vi "DB UI - Logon.vi"() -> ()   [LabVIEW 2013]
uses:
  Controls/Combo Box.ctl
  Controls/DB - Logon Extra Info.ctl
  Controls/DB - Logon Info.ctl
  <vilib>/Utility/miscctls.llb/LVComboBoxStrsAndValuesArrayTypeDef.ctl
  Controls/Logon - Enum.ctl
  Controls/DB - Logon Authentication Enum.ctl
  Controls/Global CMS.vi
  Controls/Global AMS.vi
  Controls/Global SRTRS.vi
  <vilib>/addons/database/Connection.llb/DB Tools Open Connec (String).vi
  <vilib>/addons/database/Connection.llb/Conn Execute.vi
  <vilib>/addons/database/Recordset.llb/Rec Fetch Recordset Data (R).vi
  <vilib>/addons/database/Recordset.llb/Rec Destroy - Connection.vi
  <vilib>/addons/database/Recordset.llb/Rec Fetch String Data (R).vi
  <vilib>/addons/database/NI_Database_API.lvlib
  <vilib>/Utility/miscctls.llb/LVPointTypeDef.ctl
panel:
  in  "Simulate DB Fail":bool
  out "DB available":bool
  in  "Main Application Directory (SRTRS/CMS/AMS)":path
  out "MHandler":errorcluster
  out "[IsUnicode]":bool[](array[boolean])
  out "User Has Access":bool
  out "[Stations]":string[](array[string])
  out "[AllStations]":bool
  in  "DB.Config.UserStationAccess":string="SRTRS.Config.UserStationAccess"
  out "2D data":string[][](array[string])
  in  "Overwrite HostName [ClientName] (Testing)":string
  out "Station Description":string
  out "[ClientName] Found":bool
  out "Logon":T1
  out "Logon Extra":T2
  out "Logon OK":bool
  out "[RawDataReport]":bool
  out "[TabUserAccess]":bool[](array[boolean])
  in  "Application":string
  out "DB Error":errorcluster
  out "[SpecialPrivilege] List":string[][](array[string])
  out "Logon Error":errorcluster
  in  "DB.Config.TabUserAccess":string="SRTRS.Config.TabUserAccess"
  out "[DefaultLanguage]":string
  in  "SRTRS.Config.System":string="SRTRS.Config.System"
  in  "Reinehold":bool
  out "[UserName]":string
  out "Logon PASS":bool
  in  "DB.Admin.Users":string="SRTRS.Admin.Users"
  in  "AD Simulate":T3(ring)=enum."Disable Simulation"
  out "Plant Description":string
  out "SQL":string[](array[string])
  out "[PlantId]":string
  out "[StationId]":string
  out "Initialize":bool
  out "Hostname [ClientName]":string
  in  "DB.Config.Parameter":string="SRTRS.Config.Parameter"
  in  "DB.Config.Plant":string="SRTRS.Config.Plant"
  out "Error Out":errorcluster
  in  "DB.Config.Language":string="SRTRS.Config.Language"
  in  "DB.Config.Domain":string="SRTRS.Config.Domain"
  in  "SRTRS.Config.StationSysRelation":string="SRTRS.Config.StationSysRelation"
  in  "DB.Config.Station":string="SRTRS.Config.Station"
  out "Connection Information":T4={"Connection "="SQL Server 32bit HPEnvy", "Username"="admin", "Password"="admin123"}
  out "AD available":bool
  out "Language (long form)":string
  in  "Logon Button":bool caption="Material New"
  in  "Station":T5
  in  "Plant":T5
  in  "Language":T5="English"
  in  "Domain":T5
  in  "Password":string
  in  "User":string
  # "Variables to be passed to calling VI (Must have same Label)"
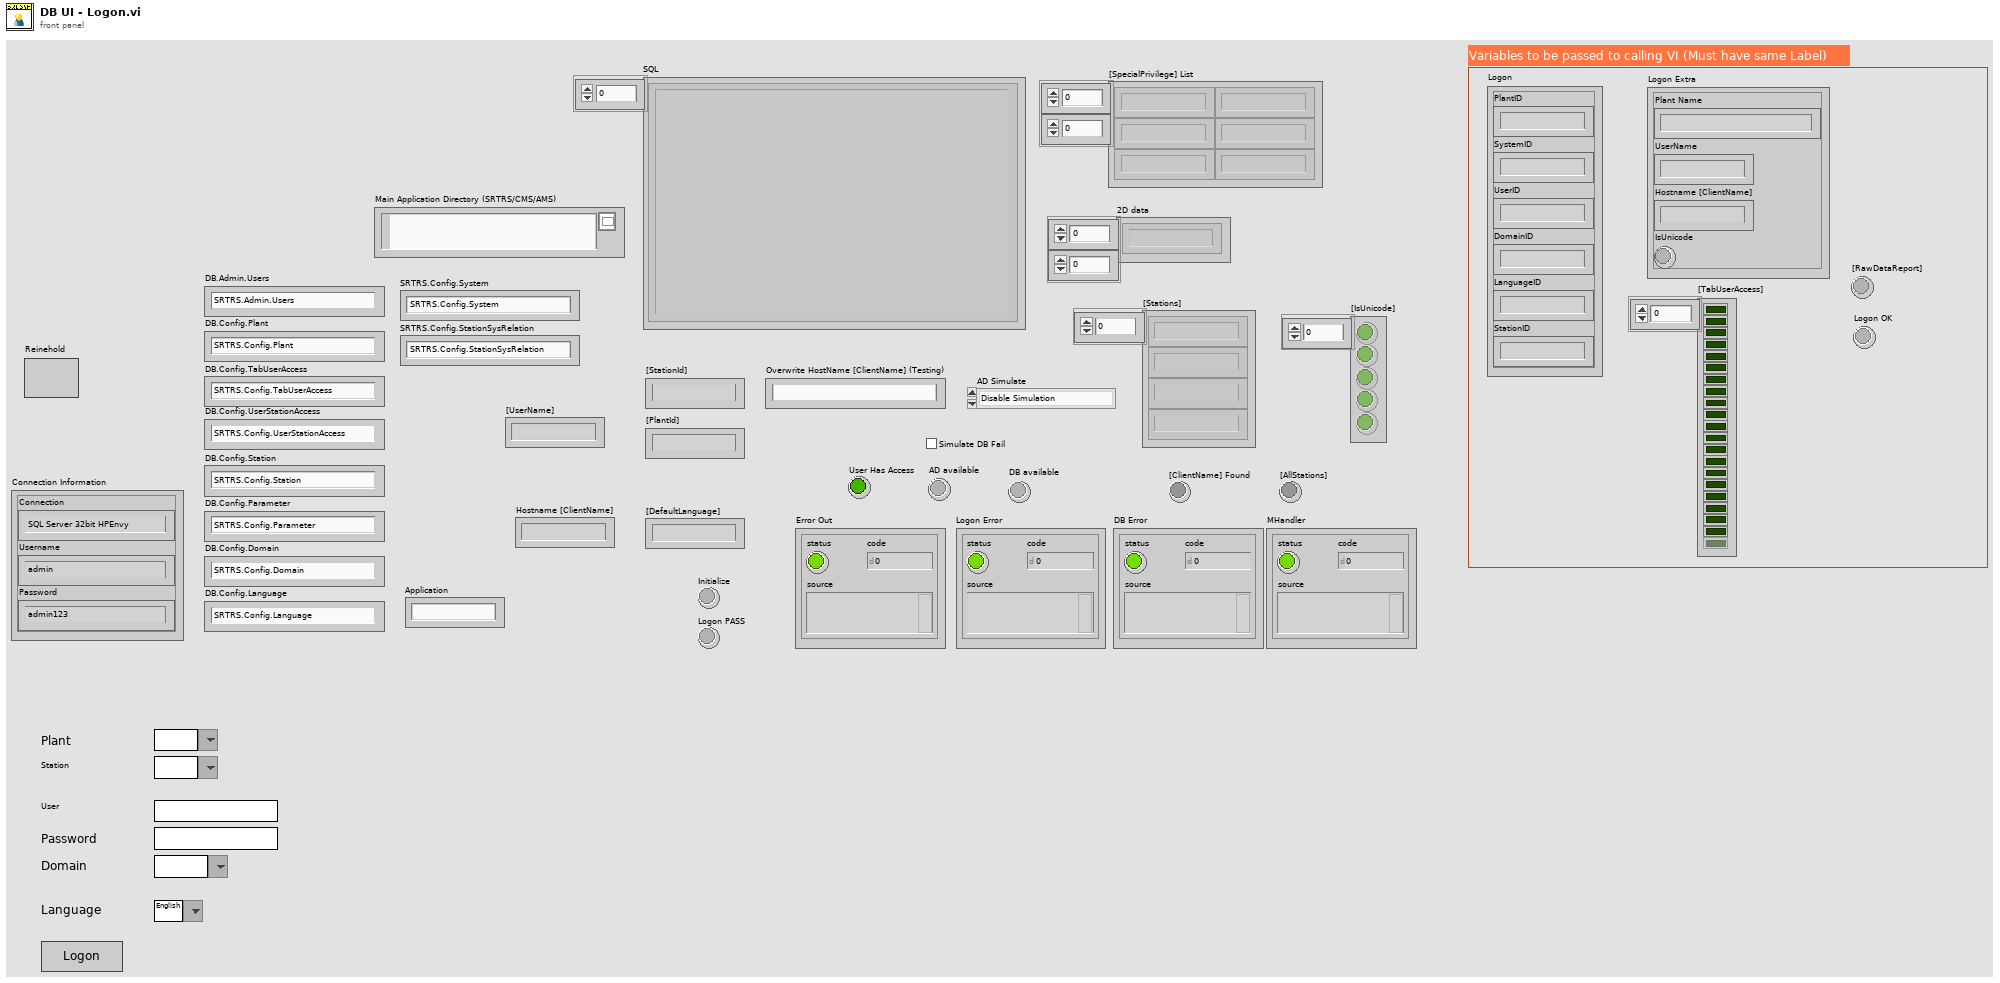
[diagram p1: front panel]
types:
  T1 = typedef "DB - Logon Info.ctl" = cluster{"PlantID":string, "SystemID":string, "UserID":string, "DomainID":string, "LanguageID":string, "StationID":string}
  T2 = typedef "DB - Logon Extra Info.ctl" = cluster{"Plant Name":string, "UserName":string, "Hostname [ClientName]":string, "IsUnicode":bool}
  T3 = enum16{"Simulate AD Available", "Simulate AD NOT Available", "Disable Simulation"}
  T4 = cluster{"Connection ":string, "Username":string, "Password":string}
  T5 = typedef "Combo Box.ctl" = string
  T6 = typedef "LVComboBoxStrsAndValuesArrayTypeDef.ctl" = cluster{"String":string, "Value":string}[]
  T7 = typedef "LVPointTypeDef.ctl" = cluster{"Horizontal":i16, "Vertical":i16}
  T8 = typedef "Connection Information Cluster.ctl" = cluster{"Connection ":string, "Username":string, "Password":string}
  T9 = typedef "NI_Database_API.lvlib/Conn ObjectReference.ctl" = refnum<k1>
  T10 = typedef "Logon - Enum.ctl" = enum16{"PC username", "PC username INFO", "Hostname", "Check AD", "Logon", "QUIT"}
  T11 = typedef "DB - Logon Authentication Enum.ctl" = enum16{"AD Authentication", "Local Authentication", "NO Authentication", "NODB Authentication"}
  T12 = typedef "DB - DB.Schema.Table.ctl" = cluster{"DB":string, "Schema":string, "Table":string}
  T13 = typedef "NI_Database_API.lvlib/Rec ObjectReference.ctl" = refnum<k1>
  T14 = cluster{"PC username":string, "Domain":string, "AD available":bool, "Username FOUND":bool, "Logon Full Name":string}
  T15 = typedef "eventvkey.ctl" = enum16{"ASCII", "Enter", "Return", "Shift", "Ctrl", "Alt", "Cmd", "Opt", "Caps", "NumLock", "Clear", "Break", "Up", "Down", "Left", "Right", "Insert", "Delete", "Home", "End", "PageUp", "PageDown", "Escape", "Help", "Pause", "ScrollLock", "F1", "F2", "F3", "F4", "F5", "F6", "F7", "F8", "F9", "F10", "F11", "F12", "F13", "F14", "F15", "F16", "F17", "F18", "F19", "F20", "F21", "F22", "F23", "F24", "Play", "VolumeUp", "VolumeDown", "Mute", "Two Byte Char"}
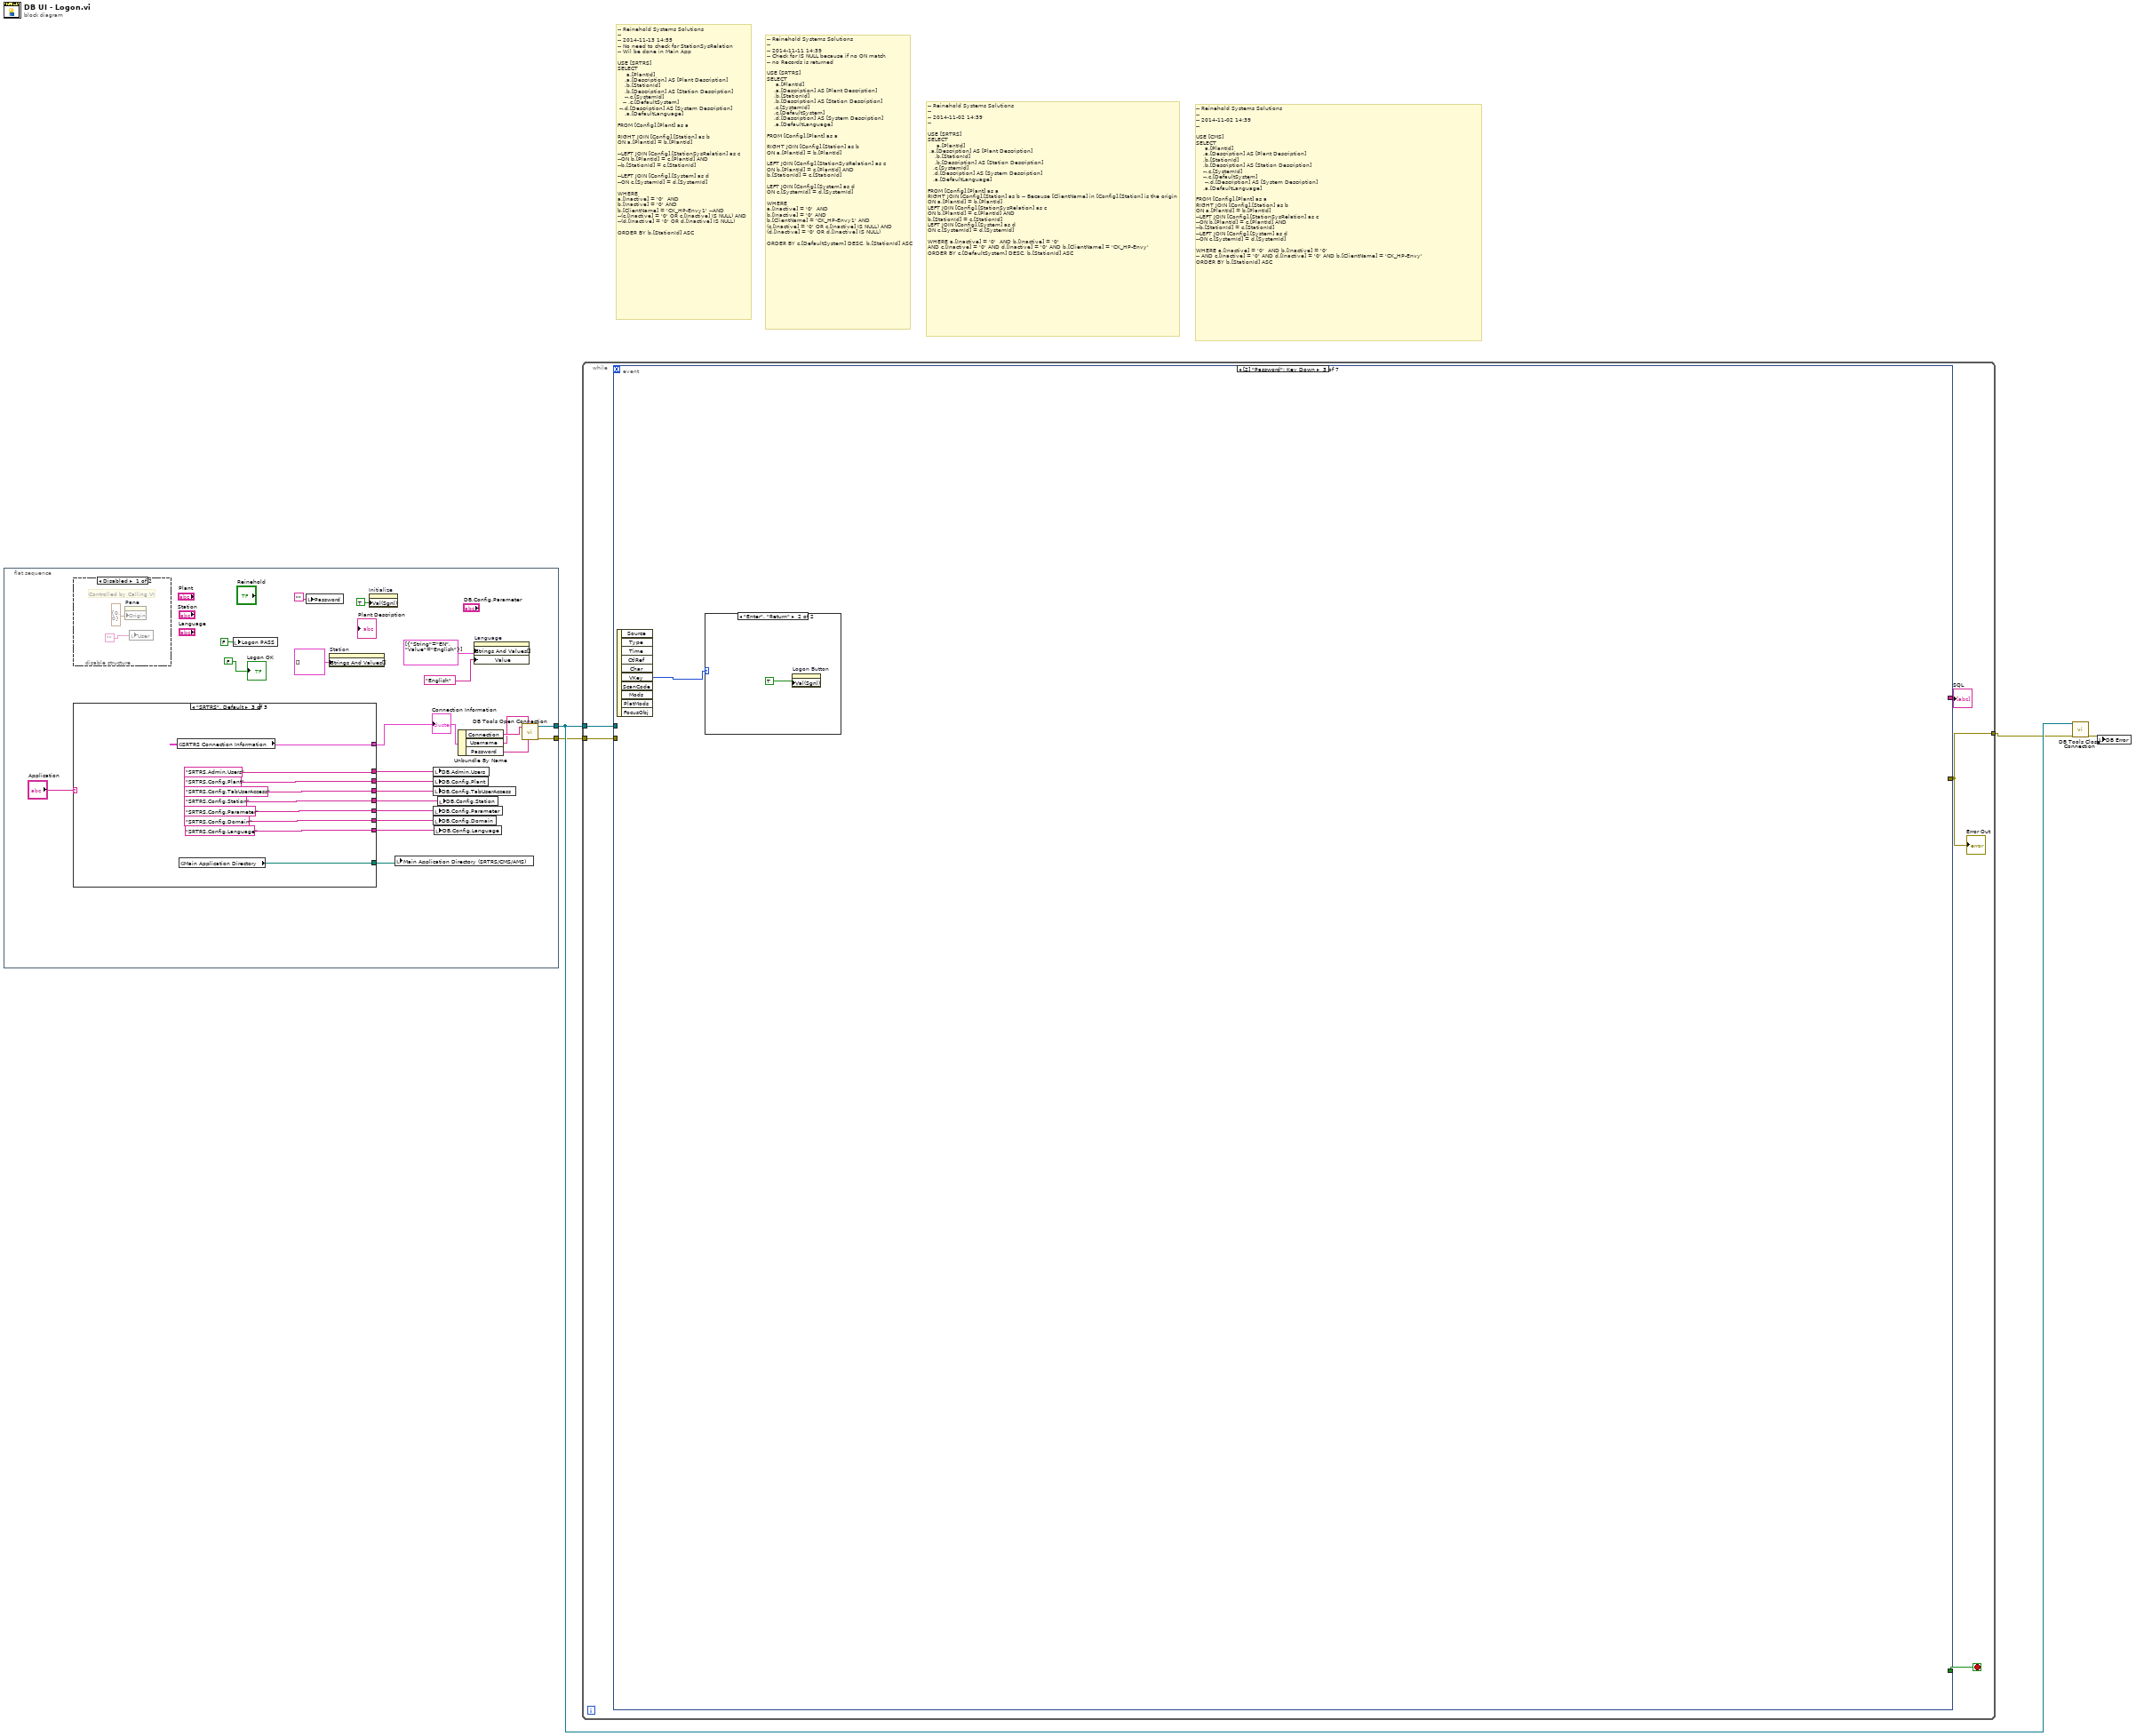
[diagram p0: block diagram]
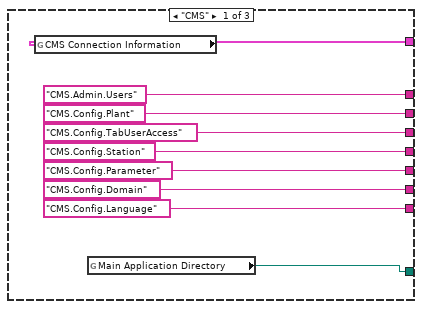
[diagram p3: hidden frame]
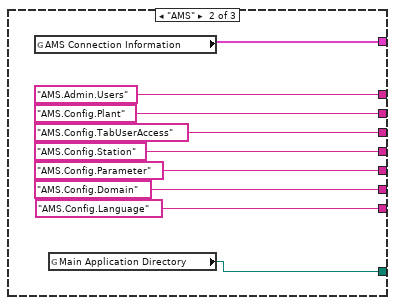
[diagram p4: hidden frame]
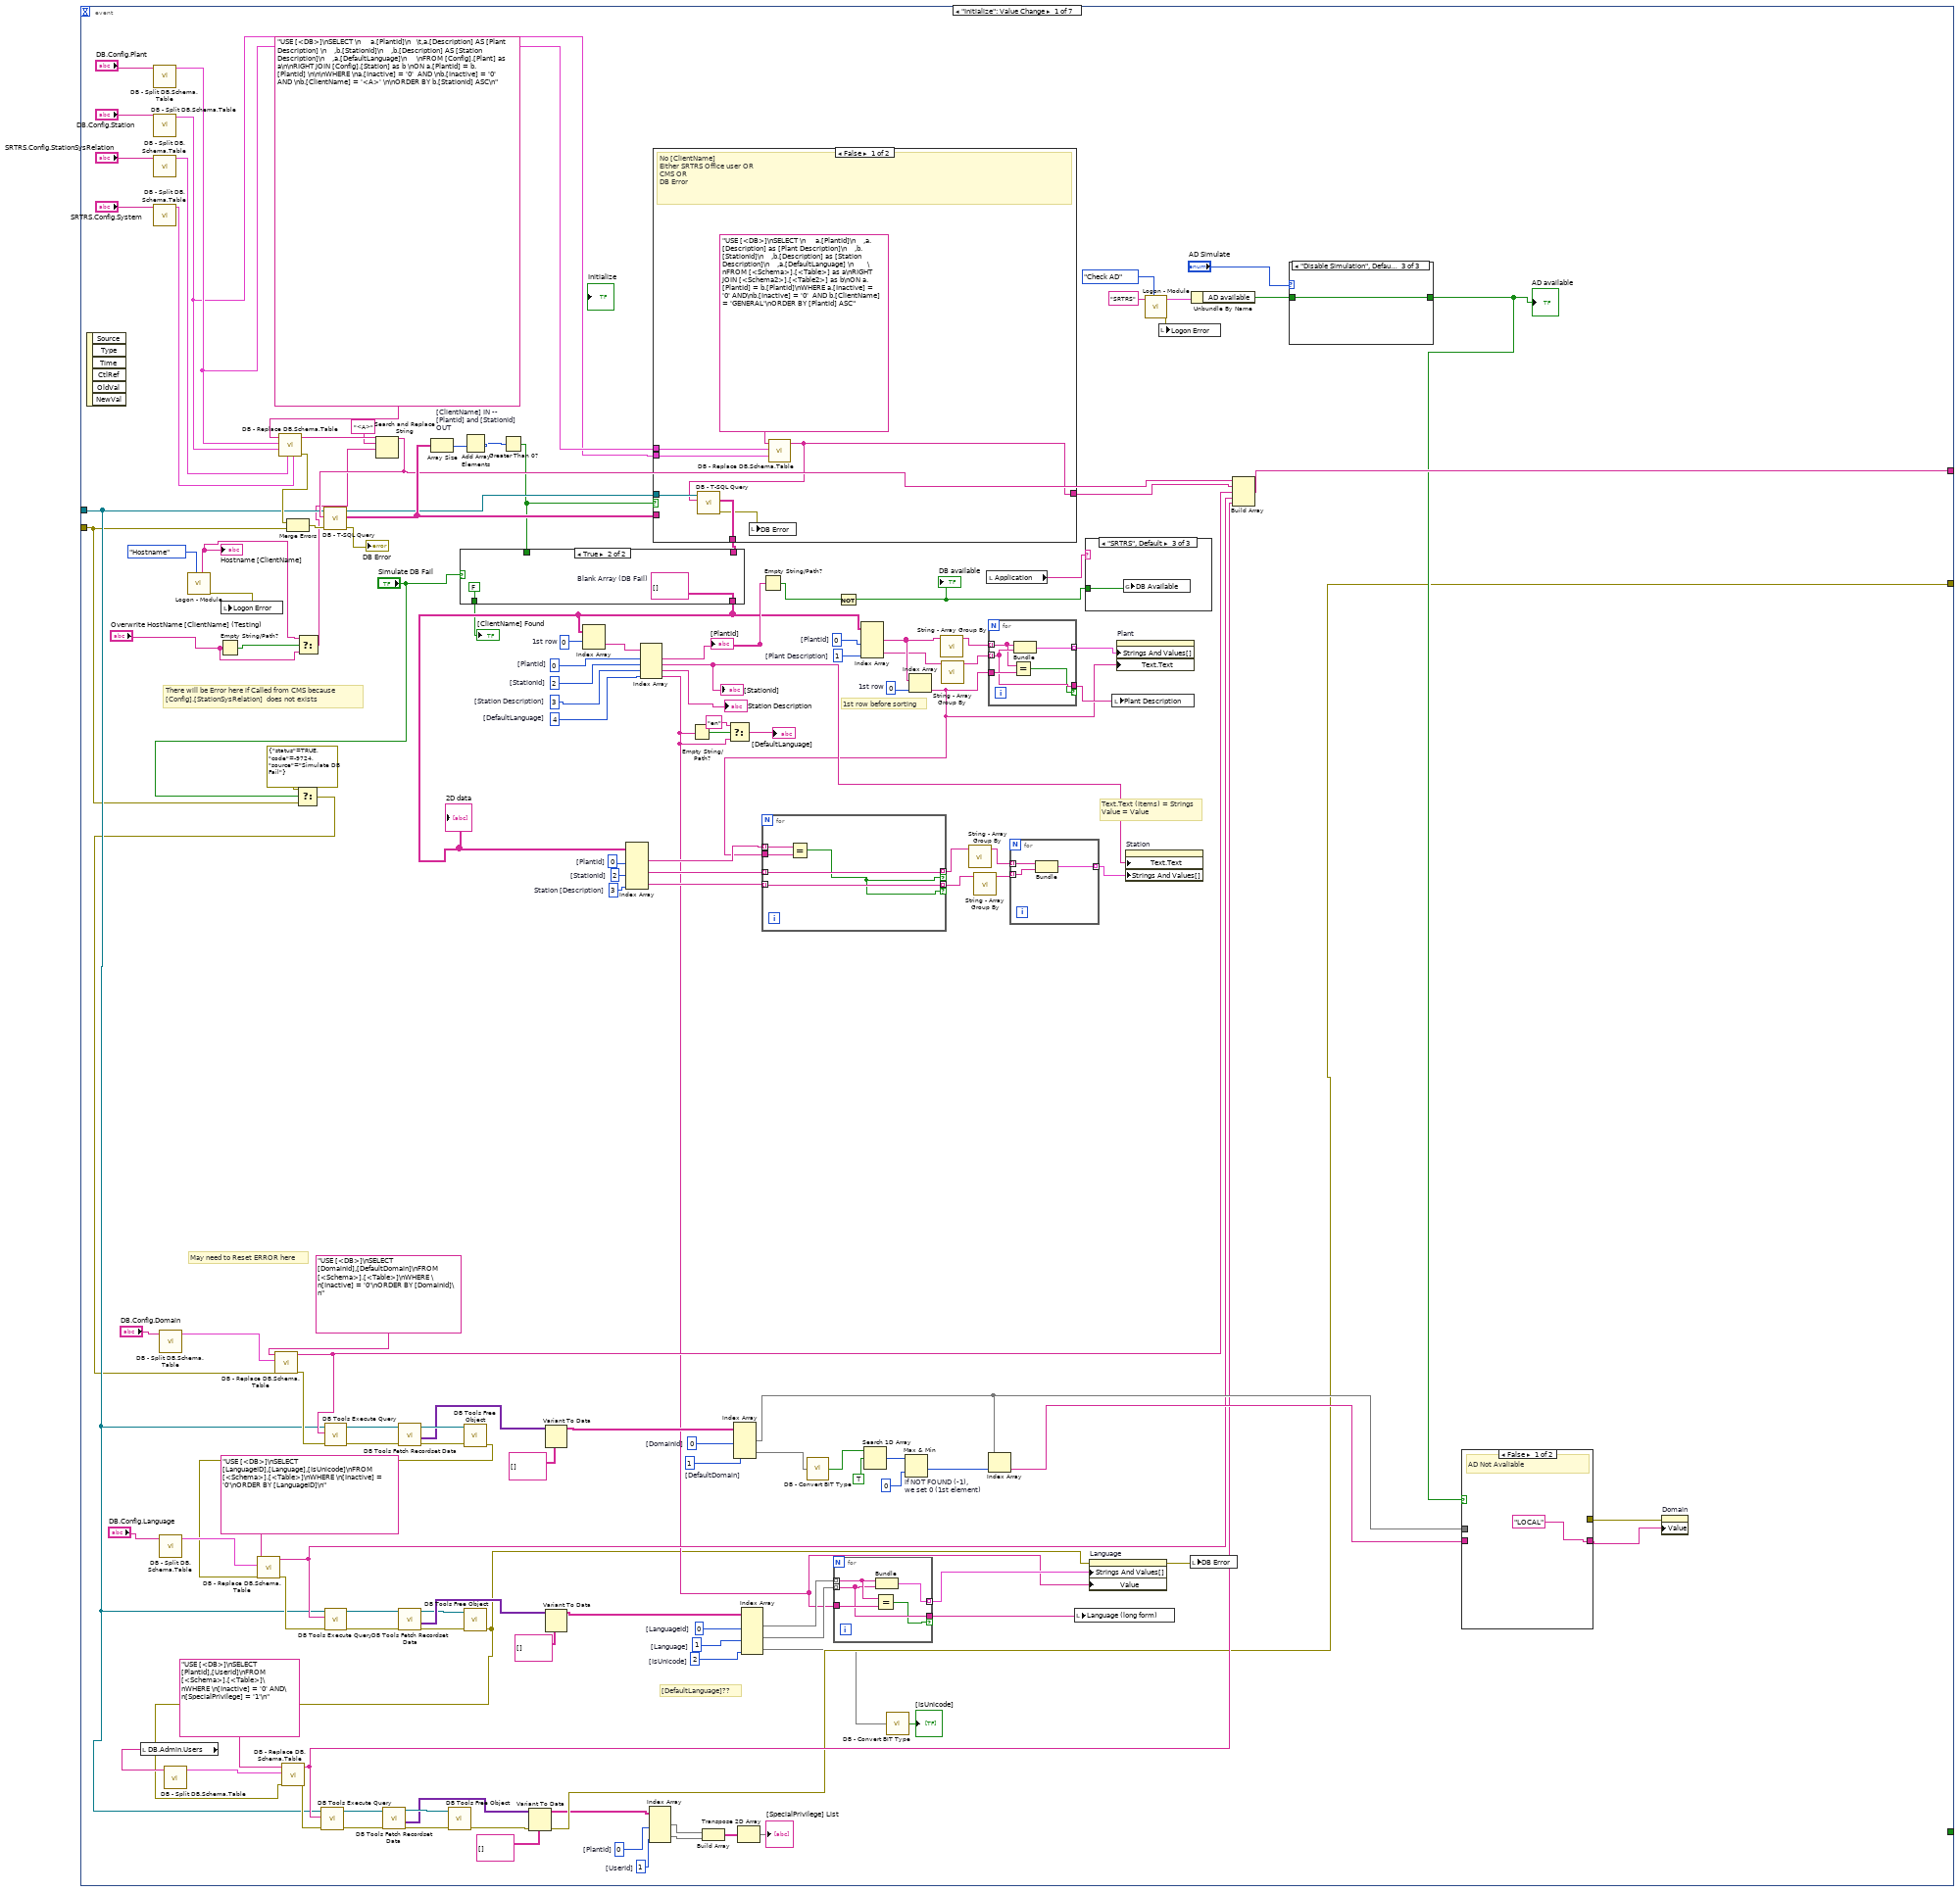
[diagram p5: hidden frame]
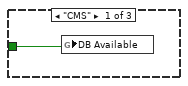
[diagram p7: hidden frame]
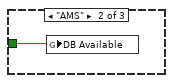
[diagram p8: hidden frame]
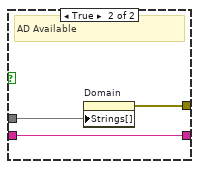
[diagram p10: hidden frame]
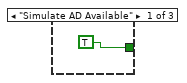
[diagram p11: hidden frame]
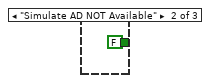
[diagram p12: hidden frame]
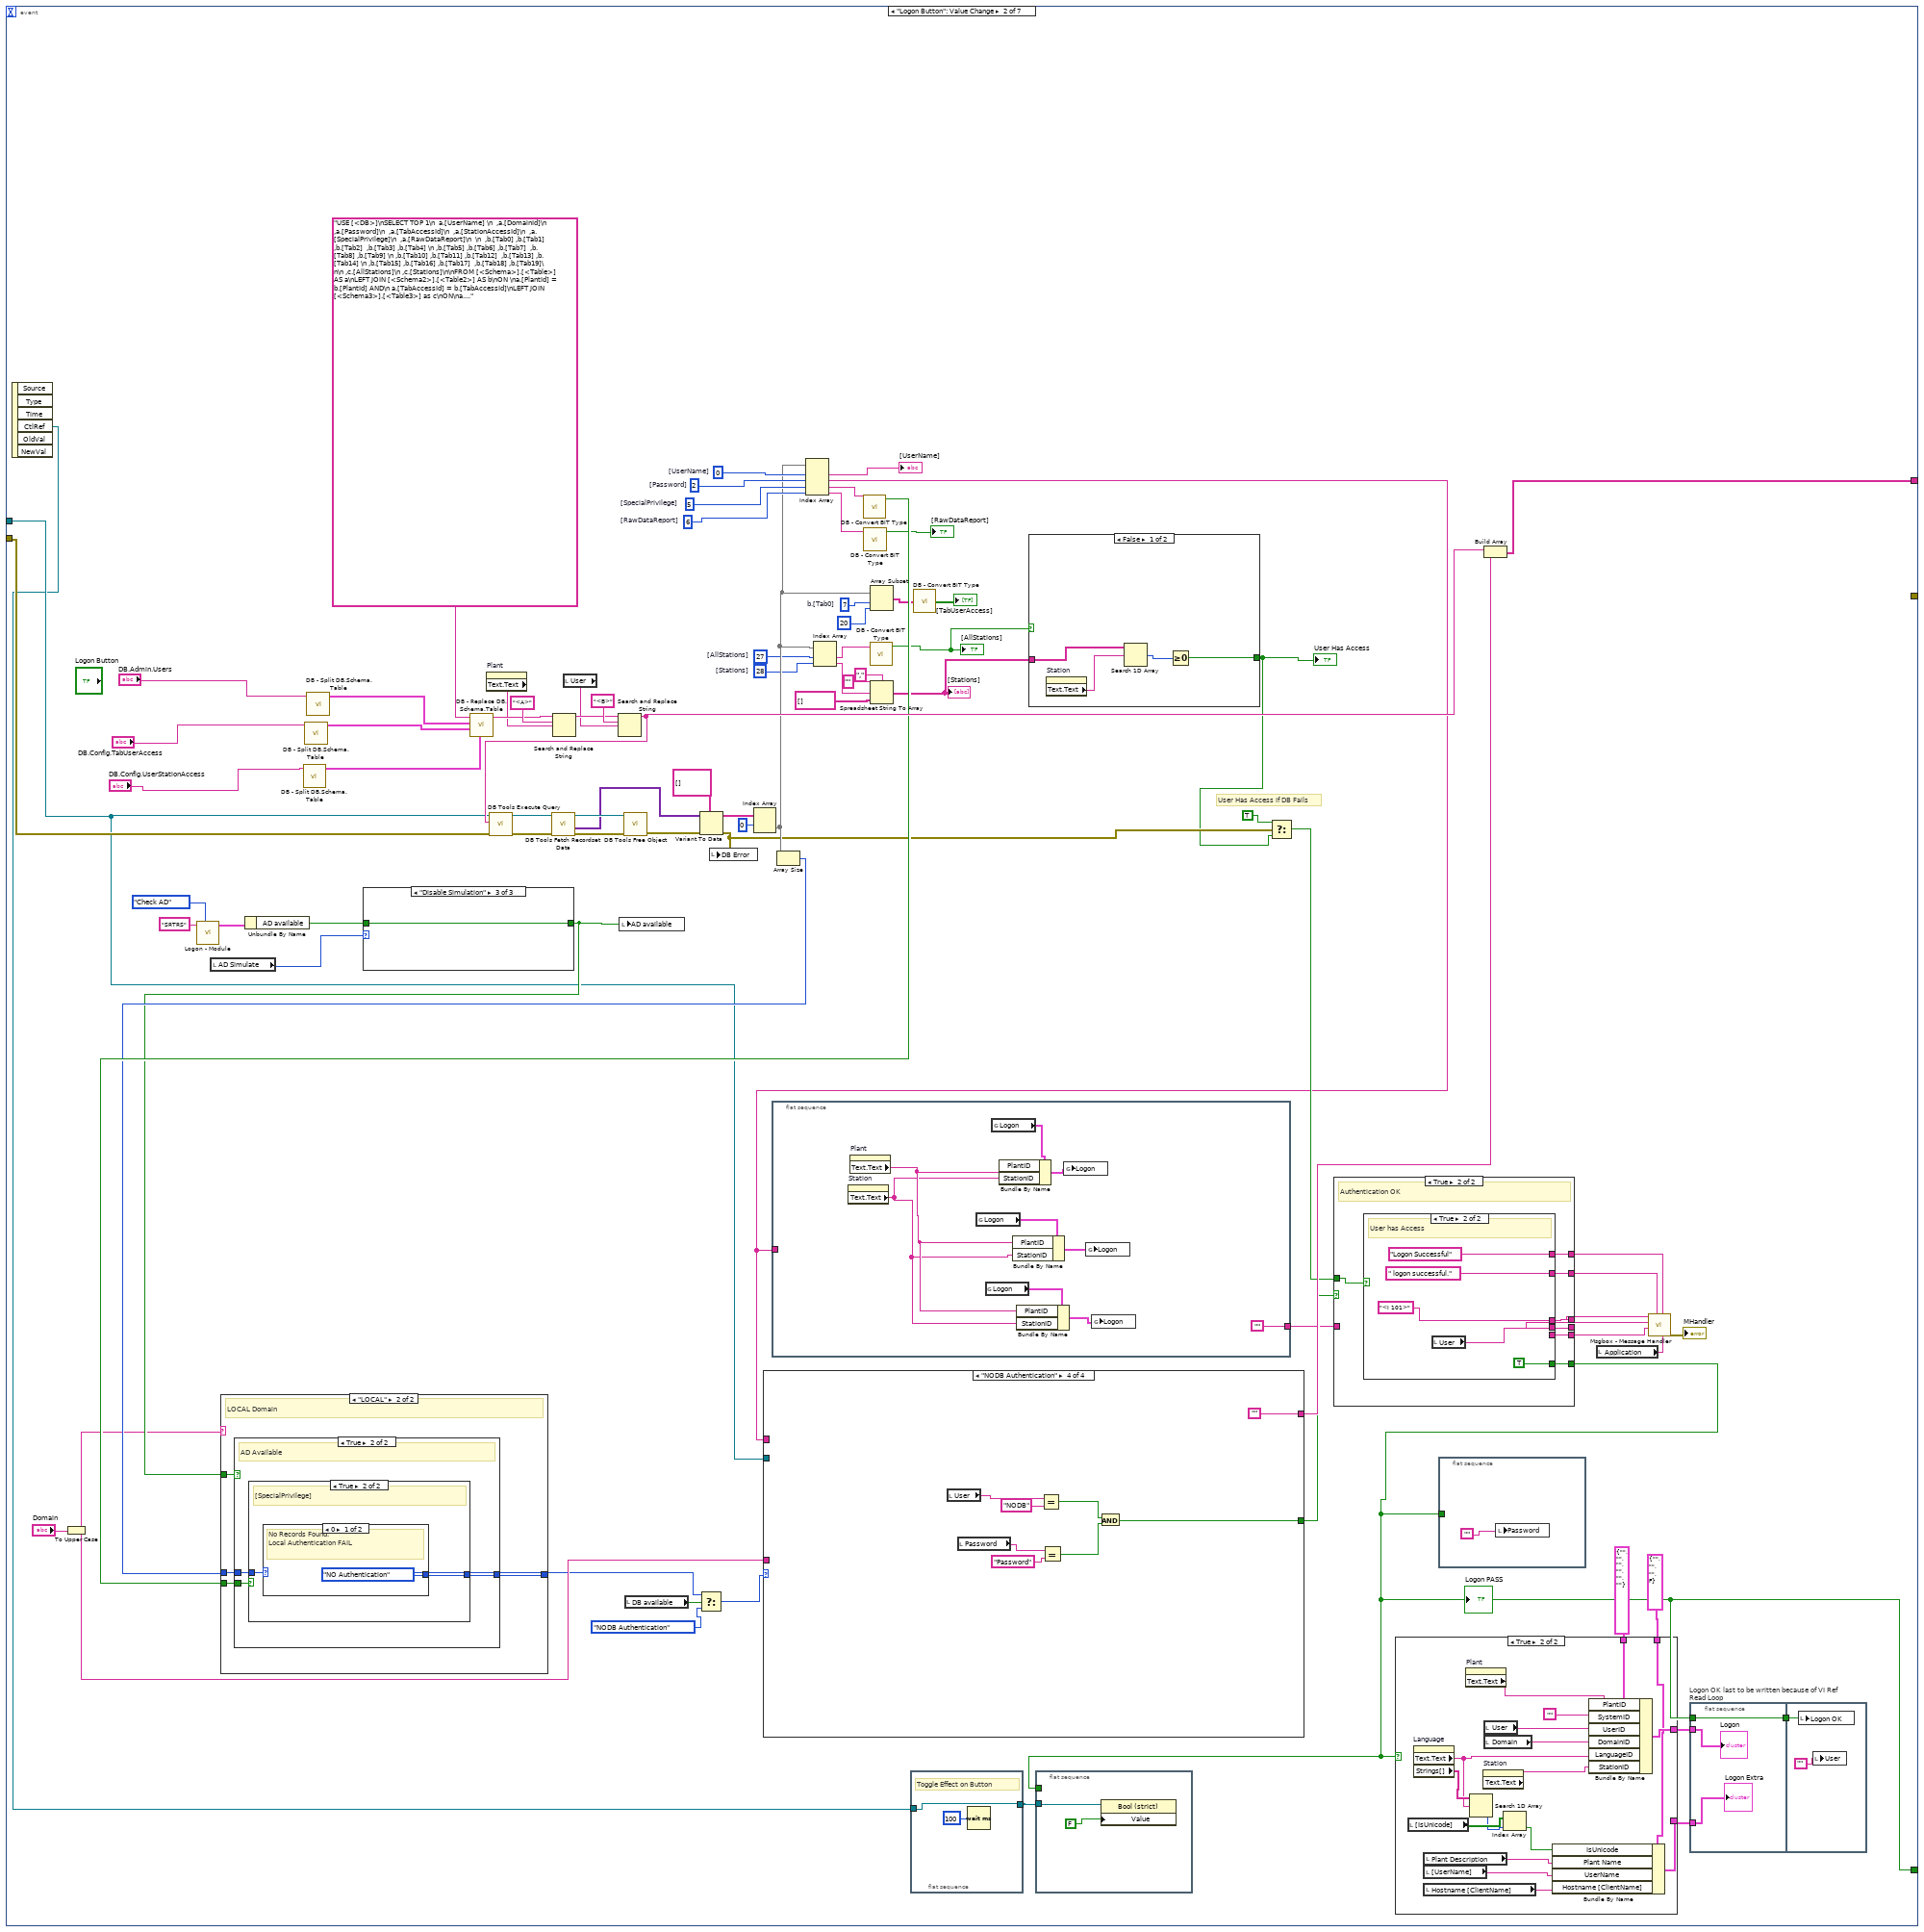
[diagram p13: hidden frame]
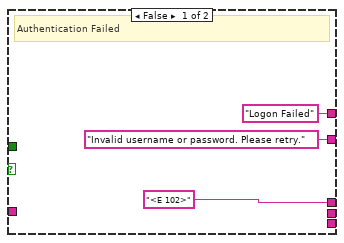
[diagram p14: hidden frame]
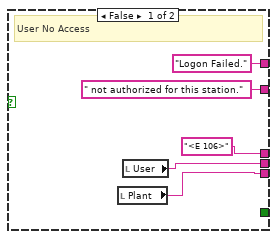
[diagram p15: hidden frame]
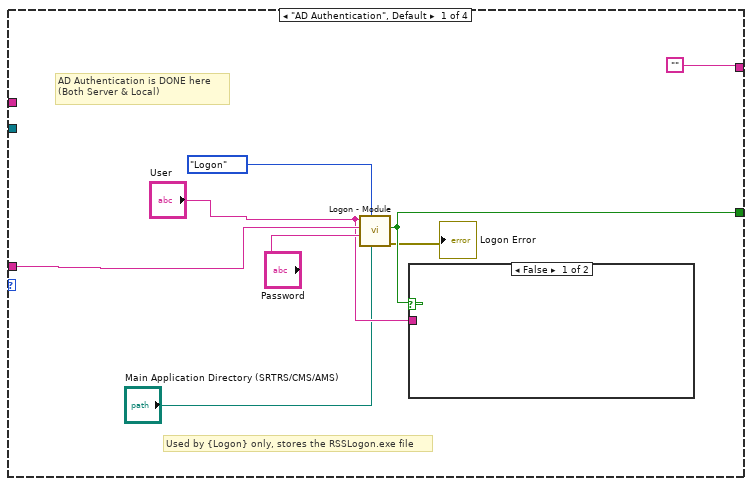
[diagram p18: hidden frame]
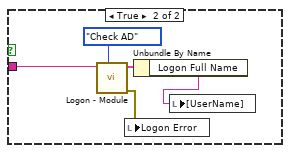
[diagram p19: hidden frame]
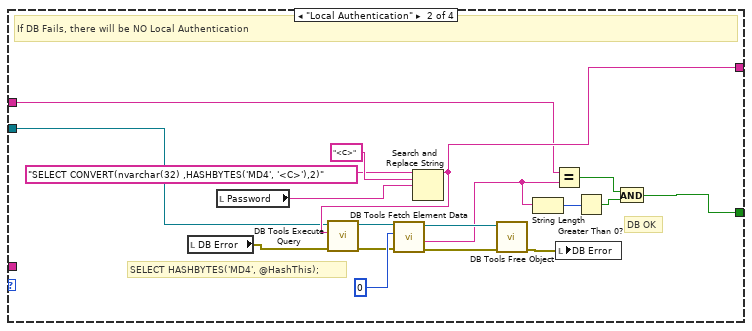
[diagram p20: hidden frame]
diagram:
  # "-- Reinehold Systems Solutions\n--\n-- 2014-11-13 14:55\n-- No need to check for StationSysRelation\n-- Wil be done in Main App\n\nUSE [SRTRS]\nSELECT \n     a.[PlantId]\n   \t,a.[Description] AS [Plant Description] \n    ,b.[StationId]\n    ,b.[Description] AS [Station Description]\n   \t--,c.[SystemId]\n   -- ,c.[DefaultSystem]\n\t--,d.[Description] AS [System Description]\n    ,a.[DefaultLanguage]\n     \nFROM [Config].[Plant] as a\n\nRIGHT JOIN [Config].[Station] as b \nON a.[PlantId] = b.[PlantId] \n\n--LEFT JOIN [Config].[StationSysRelation] as c\n--ON b.[PlantId] = c.[PlantId] AND\n--b.[StationId] = c.[StationId] \n\n--LEFT JOIN [Config].[System] as d\n--ON c.[SystemId] = d.[SystemId] \n \nWHERE \na.[Inactive] = '0'  AND \nb.[Inactive] = '0' AND \nb.[ClientName] = 'CK_HP-Envy1' --AND\n--(c.[Inactive] = '0' OR c.[Inactive] IS NULL) AND \n--(d.[Inactive] = '0' OR d.[Inactive] IS NULL)  \n\nORDER BY b.[StationId] ASC"
  # "-- Reinehold Systems Solutions\n--\n-- 2014-11-11 14:39\n-- Check for IS NULL because if no ON match\n-- no Records is returned\n\nUSE [SRTRS]\nSELECT \n     a.[PlantId]\n   \t,a.[Description] AS [Plant Description] \n    ,b.[StationId]\n    ,b.[Description] AS [Station Description]\n   \t,c.[SystemId]\n    ,c.[DefaultSystem]\n\t   ,d.[Description] AS [System Description]\n    ,a.[DefaultLanguage]\n     \nFROM [Config].[Plant] as a\n\nRIGHT JOIN [Config].[Station] as b \nON a.[PlantId] = b.[PlantId] \n\nLEFT JOIN [Config].[StationSysRelation] as c\nON b.[PlantId] = c.[PlantId] AND\nb.[StationId] = c.[StationId] \n\nLEFT JOIN [Config].[System] as d\nON c.[SystemId] = d.[SystemId] \n \nWHERE \na.[Inactive] = '0'  AND \nb.[Inactive] = '0' AND \nb.[ClientName] = 'CK_HP-Envy1' AND\n(c.[Inactive] = '0' OR c.[Inactive] IS NULL) AND \n(d.[Inactive] = '0' OR d.[Inactive] IS NULL)  \n\nORDER BY c.[DefaultSystem] DESC, b.[StationId] ASC"
  # "-- Reinehold Systems Solutions\n--\n-- 2014-11-02 14:39\n--\n\nUSE [CMS]\nSELECT \n     a.[PlantId]\n   \t,a.[Description] AS [Plant Description] \n    ,b.[StationId]\n    ,b.[Description] AS [Station Description]\n   \t--,c.[SystemId]\n    --,c.[DefaultSystem]\n\t    --,d.[Description] AS [System Description]\n    ,a.[DefaultLanguage]\n\nFROM [Config].[Plant] as a\nRIGHT JOIN [Config].[Station] as b \nON a.[PlantId] = b.[PlantId]\n--LEFT JOIN [Config].[StationSysRelation] as c\n--ON b.[PlantId] = c.[PlantId] AND\n--b.[StationId] = c.[StationId]\n--LEFT JOIN [Config].[System] as d\n--ON c.[SystemId] = d.[SystemId]\n\nWHERE a.[Inactive] = '0'  AND b.[Inactive] = '0' \n-- AND c.[Inactive] = '0' AND d.[Inactive] = '0' AND b.[ClientName] = 'CK_HP-Envy'\nORDER BY b.[StationId] ASC"
  # "-- Reinehold Systems Solutions\n--\n-- 2014-11-02 14:39\n--\n\nUSE [SRTRS]\nSELECT \n     a.[PlantId]\n\t,a.[Description] AS [Plant Description] \n    ,b.[StationId]\n    ,b.[Description] AS [Station Description]\n  \t,c.[SystemId]\n  \t,d.[Description] AS [System Description]\n   ,a.[DefaultLanguage]\n     \nFROM [Config].[Plant] as a\nRIGHT JOIN [Config].[Station] as b -- Because [ClientName] in [Config].[Station] is the origin\nON a.[PlantId] = b.[PlantId]\nLEFT JOIN [Config].[StationSysRelation] as c\nON b.[PlantId] = c.[PlantId] AND\nb.[StationId] = c.[StationId]\nLEFT JOIN [Config].[System] as d\nON c.[SystemId] = d.[SystemId]\n \nWHERE a.[Inactive] = '0'  AND b.[Inactive] = '0' \nAND c.[Inactive] = '0' AND d.[Inactive] = '0' AND b.[ClientName] = 'CK_HP-Envy'\nORDER BY c.[DefaultSystem] DESC, b.[StationId] ASC"
  n1 = flat-sequence {
    tunnel: [w23] -> w4
    tunnel: [w7] -> w3
    frame #0 {
      n2 = case shown="\"SRTRS\", Default" "Application" {
        tunnel: [w37 w39 w55] -> w19
        tunnel: ["CMS.Admin.Users" ("DB.Schema.Table\n(SRTRS.Admin.Users)") "AMS.Admin.Users" ("DB.Schema.Table\n(SRTRS.Admin.Users)") "SRTRS.Admin.Users" ("DB.Schema.Table\n(SRTRS.Admin.Users)")] -> w18
        tunnel: ["CMS.Config.Plant" ("DB.Schema.Table\nDB.Config.Plant") "AMS.Config.Plant" ("DB.Schema.Table\nDB.Config.Plant") "SRTRS.Config.Plant" ("DB.Schema.Table\nDB.Config.Plant")] -> w17
        tunnel: ["CMS.Config.TabUserAccess" ("DB.Config.TabUserAccess") "AMS.Config.TabUserAccess" ("DB.Config.TabUserAccess") "SRTRS.Config.TabUserAccess" ("DB.Config.TabUserAccess")] -> w16
        tunnel: ["CMS.Config.Station" ("SRTRS.Config.Station") "AMS.Config.Station" ("SRTRS.Config.Station") "SRTRS.Config.Station" ("SRTRS.Config.Station")] -> w15
        tunnel: ["CMS.Config.Parameter" ("DB.Config.Parameter") "AMS.Config.Parameter" ("DB.Config.Parameter") "SRTRS.Config.Parameter" ("DB.Config.Parameter")] -> w14
        tunnel: ["CMS.Config.Domain" ("DB.Config.Domain") "AMS.Config.Domain" ("DB.Config.Domain") "SRTRS.Config.Domain" ("DB.Config.Domain")] -> w13
        tunnel: ["CMS.Config.Language" ("DB.Config.TabUserAccess") "AMS.Config.Language" ("DB.Config.TabUserAccess") "SRTRS.Config.Language" ("DB.Config.TabUserAccess")] -> w12
        tunnel: [w29 w38 w47] -> w8
        frame "CMS" {
          n3 = global read "Global CMS.vi" "CMS Connection Information"() -> (w37:T8)
          n4 = global read "Global CMS.vi" "Main Application Directory"() -> (w29:path)
        }
        frame "AMS" {
          n5 = global read "Global AMS.vi" "AMS Connection Information"() -> (w39:T8)
          n6 = global read "Global AMS.vi" "Main Application Directory"() -> (w38:path)
        }
        frame "SRTRS", Default {
          n7 = global read "Global SRTRS.vi" "SRTRS Connection Information"() -> (w55:T8)
          n8 = global read "Global SRTRS.vi" "Main Application Directory"() -> (w47:path)
        }
      }
      "Connection Information" <- w19
      n9 = disable-structure shown="Disabled" {
        frame Disabled {
          # "Controlled by Calling VI"
          n10 = property on="Pane" class="Pane"("Origin"=T7 {"Horizontal"=0, "Vertical"=0}) -> ()  [unwired: 2 in, 2 out]
          n11 = local write "User"("") -> ()
        }
        frame Enabled {
        }
      }
      n12 = local write "Logon PASS"(FALSE ("Logon PASS")) -> ()
      n13 = local write "Password"("") -> ()
      n14 = property on="Station" class="CmbBox (strict)"("Strings And Values[]"=T6 [] ("Strings And Values []")) -> ()  [unwired: 2 in, 2 out]
      n15 = property on="Initialize" class="Bool (strict)"("Val(Sgnl)"=TRUE ("Value (Signaling)")) -> ()  [unwired: 2 in, 2 out]
      n16 = local write "Main Application Directory (SRTRS/CMS/AMS)"(w8) -> ()
      n17 = local write "DB.Admin.Users"(w18) -> ()
      n18 = local write "DB.Config.Plant"(w17) -> ()
      n19 = local write "DB.Config.TabUserAccess"(w16) -> ()
      n20 = local write "DB.Config.Parameter"(w14) -> ()
      n21 = local write "DB.Config.Domain"(w13) -> ()
      n22 = local write "DB.Config.Language"(w12) -> ()
      n23 = local write "DB.Config.Station"(w15) -> ()
      n24 = Unbundle By Name(w19) -> ("Connection"=w26:string, "Username"=w25:string, "Password"=w24:string)
      n25 = property on="Language" class="CmbBox (strict)"("Strings And Values[]"=T6 [{"String"="EN", "Value"="English"}] ("Strings And Values []"), "Value"=T5 "English" ("Language")) -> ()  [unwired: 2 in, 2 out]
      n26 = call-poly <vilib>:"DB Tools Open Connection.vi"("password"=w24, "userID"=w25, "connection information"=w26) -> ("error out"=w7:errorcluster, "connection reference"=w23:T9)  [unwired: 5 in]
      "Logon OK" <- FALSE ("Logon OK")
    }
  }
  n27 = while {
    tunnel: w4 -> [w59]
    tunnel: w3 -> [w58]
    tunnel: [w57] -> w2
    stop <- w60 stop-if-true
    n28 = event shown="[2] \"Password\": Key Down" {
      selector: _ -> [_ _ _ _ _ _ _]
      dyn-events: _ -> [_ _ _ _ _ _ _]
      timeout: _ -> [_ _ _ _ _ _ _]
      tunnel: [_ w259 _ _ _ _ _] -> w60
      tunnel: w59 -> [w101 w300 _ _ _ _ _]
      tunnel: w58 -> [w64 w320 _ _ _ _ _]
      tunnel: [w139 _ _ _ _ _ _] -> w57
      tunnel: [w202 w311 _ _ _ _ _] -> w56
      event "Initialize": Value Change {
        w81 = 2  # [IsUnicode]
        w84 = 0  # [PlantId]
        w93 = 3  # Station [Description]
        w99 = 2  # [StationId]
        w115 = 0  # 1st row
        w110 = 1  # [Plant Description]
        w109 = 0  # [PlantId]
        w135 = 1  # [UserId]
        w136 = 0  # [PlantId]
        w149 = 4  # [DefaultLanguage]
        w153 = 0  # 1st row
        w150 = 3  # [Station Description]
        w169 = 1  # [Language]
        w172 = 0  # [LanguageId]
        w192 = 1  # [DefaultDomain]
        w191 = 0  # [DomainId]
        w151 = 2  # [StationId]
        w152 = 0  # [PlantId]
        w208 = "USE [<DB>]\nSELECT \n     a.[PlantId]\n   \t,a.[Description] AS [Plant Description] \n    ,b.[StationId]\n    ,b.[Description] AS [Station Description]\n    ,a.[DefaultLanguage]\n     \nFROM [Config].[Plant] as a\n\nRIGHT JOIN [Config].[Station] as b \nON a.[PlantId] = b.[PlantId] \n\n\nWHERE \na.[Inactive] = '0'  AND \nb.[Inactive] = '0' AND \nb.[ClientName] = '<A>' \n\nORDER BY b.[StationId] ASC\n"  # [ClientName] IN --  [PlantId] and [StationId] OUT
        # "There will be Error here if Called from CMS because \n[Config].[StationSysRelation]  does not exists"
        # "1st row before sorting"
        # "May need to Reset ERROR here"
        # "Text.Text (Items) = Strings\nValue = Value"
        # "[DefaultLanguage]??"
        n29 = event-data() -> ()  [unwired: 1 in, 6 out]
        n30 = local read "DB.Admin.Users"() -> (w148:string)
        n31 = call "DB - Split DB.Schema.Table.vi"("DB.Schema.Table"="DB.Config.Plant") -> ("DB.Schema.Table"=w105:T12)  [unwired: 10 in]
        n32 = call "DB - Split DB.Schema.Table.vi"("DB.Schema.Table"="DB.Config.Station") -> ("DB.Schema.Table"=w104:T12)  [unwired: 10 in]
        n33 = call "DB - Split DB.Schema.Table.vi"("DB.Schema.Table"="SRTRS.Config.StationSysRelation") -> ("DB.Schema.Table"=w103:T12)  [unwired: 10 in]
        n34 = call "DB - Split DB.Schema.Table.vi"("DB.Schema.Table"="SRTRS.Config.System") -> ("DB.Schema.Table"=w102:T12)  [unwired: 10 in]
        n35 = call "DB - Split DB.Schema.Table.vi"("DB.Schema.Table"="DB.Config.Domain") -> ("DB.Schema.Table"=w198:T12)  [unwired: 10 in]
        n36 = call "DB - Split DB.Schema.Table.vi"("DB.Schema.Table"="DB.Config.Language") -> ("DB.Schema.Table"=w173:T12)  [unwired: 10 in]
        n37 = call "DB - Split DB.Schema.Table.vi"("DB.Schema.Table"=w148) -> ("DB.Schema.Table"=w146:T12)  [unwired: 10 in]
        n38 = call "Logon - Module.vi"("Logon - Enum"=Logon_-_Enum."Hostname") -> ("Error Out"=w129:errorcluster, "Hostname"=w96:string)  [unwired: 5 in, 4 out]
        "Hostname [ClientName]" <- w96
        n39 = Empty String/Path?(string/path="Overwrite HostName [ClientName] (Testing)") -> (empty?=w97:bool)
        n40 = local write "Logon Error"(w129) -> ()
        n41 = call "DB - Replace DB.Schema.Table.vi"("DB.Schema.Table 4"=w102, "DB.Schema.Table 3"=w103, "DB.Schema.Table 2"=w104, "DB.Schema.Table"=w105, "string in"=w208) -> ("error out"=w117:errorcluster, "string out"=w207:string)  [unwired: 5 in]
        n42 = Merge Errors(w117, w64) -> (w116:errorcluster)
        n43 = Select(t=errorcluster {"status"=TRUE, "code"=-9724, "source"="Simulate DB Fail"} ("error constant"), s="Simulate DB Fail", f=w64) -> (s? t:f=w65:errorcluster)
        n44 = call "DB - Replace DB.Schema.Table.vi"("error in (no error)"=w65, "DB.Schema.Table"=w198, "string in"="USE [<DB>]\nSELECT [DomainId],[DefaultDomain]\nFROM [<Schema>].[<Table>]\nWHERE \n[Inactive] = '0'\nORDER BY [DomainId]\n") -> ("error out"=w122:errorcluster, "string out"=w154:string)  [unwired: 7 in]
        n45 = Select(t=w96, s=w97, f="Overwrite HostName [ClientName] (Testing)") -> (s? t:f=w94:string)
        n46 = call-poly <vilib>:"DB Tools Execute Query.vi"("error in (no error)"=w122, "SQL query"=w154, "connection reference"=w101) -> ("error out"=w196:errorcluster, "recordset reference"=w201:T13)  [unwired: 5 in]
        n47 = Search and Replace String(input string=w207, search string="<A>" ("input string"), replace string=w94) -> (result string=w123:string)  [unwired: 5 in, 3 out]
        n48 = call "DB - T-SQL Query.vi"("error in (no error)"=w116, "T-SQL"=w123, "connection reference"=w101) -> ("error out"=→"DB Error":errorcluster, "2D data"=w126:string[][], "connection reference"=w125:T9)  [unwired: 6 in]
        n49 = call-poly <vilib>:"DB Tools Fetch Recordset Data.vi"("error in (no error)"=w196, "recordset reference"=w201) -> ("error out"=w195:errorcluster, "recordset data"=w193:variant[][], "recordset reference out"=w200:T13)  [unwired: 3 in]
        n50 = Array Size(array=w126) -> (size(s)=w127:i32[])
        n51 = Add Array Elements(numeric array=w127) -> (sum=w106:i32)
        n52 = call-poly <vilib>:"DB Tools Free Object.vi"("error in (no error)"=w195, "recordset reference"=w200) -> ("error out"=w120:errorcluster)  [unwired: 8 in, 1 out]
        n53 = call "DB - Replace DB.Schema.Table.vi"("error in (no error)"=w120, "DB.Schema.Table"=w173, "string in"="USE [<DB>]\nSELECT [LanguageID],[Language],[IsUnicode]\nFROM [<Schema>].[<Table>]\nWHERE \n[Inactive] = '0'\nORDER BY [LanguageID]\n") -> ("error out"=w119:errorcluster, "string out"=w170:string)  [unwired: 7 in]
        n54 = call-poly <vilib>:"DB Tools Execute Query.vi"("error in (no error)"=w119, "SQL query"=w170, "connection reference"=w101) -> ("error out"=w178:errorcluster, "recordset reference"=w175:T13)  [unwired: 5 in]
        n55 = call-poly <vilib>:"DB Tools Fetch Recordset Data.vi"("error in (no error)"=w178, "recordset reference"=w175) -> ("error out"=w179:errorcluster, "recordset data"=w181:variant[][], "recordset reference out"=w176:T13)  [unwired: 3 in]
        n56 = call-poly <vilib>:"DB Tools Free Object.vi"("error in (no error)"=w179, "recordset reference"=w176) -> ("error out"=w62:errorcluster)  [unwired: 8 in, 1 out]
        n57 = call "DB - Replace DB.Schema.Table.vi"("error in (no error)"=w62, "DB.Schema.Table"=w146, "string in"="USE [<DB>]\nSELECT [PlantId],[UserId]\nFROM [<Schema>].[<Table>]\nWHERE \n[Inactive] = '0' AND\n[SpecialPrivilege] = '1'\n") -> ("error out"=w121:errorcluster, "string out"=w145:string)  [unwired: 7 in]
        n58 = call-poly <vilib>:"DB Tools Execute Query.vi"("error in (no error)"=w121, "SQL query"=w145, "connection reference"=w101) -> ("error out"=w128:errorcluster, "recordset reference"=w140:T13)  [unwired: 5 in]
        n59 = call-poly <vilib>:"DB Tools Fetch Recordset Data.vi"("error in (no error)"=w128, "recordset reference"=w140) -> ("error out"=w143:errorcluster, "recordset data"=w141:variant[][], "recordset reference out"=w144:T13)  [unwired: 3 in]
        n60 = call-poly <vilib>:"DB Tools Free Object.vi"("error in (no error)"=w143, "recordset reference"=w144) -> ("error out"=w138:errorcluster)  [unwired: 8 in, 1 out]
        n61 = Greater Than 0?(x=w106) -> (x > 0?=w68:bool)
        n62 = Variant To Data(error in=w138, type=string[][] [], Variant=w141) -> (data=w137:string[][], error out=w139:errorcluster)
        n63 = Variant To Data(type=string[][] [], Variant=w193) -> (data=w190:string[][])  [unwired: 1 in, 1 out]
        n64 = Variant To Data(type=string[][] [], Variant=w181) -> (data=w171:string[][])  [unwired: 1 in, 1 out]
        n65 = Index Array(array=w137, index (col) #1=w136, index (col) #2=w135) -> (element #1=w134:string[], element #2=w133:string[])  [unwired: 2 in]
        n66 = case shown="False" w68 {
          tunnel: w126 -> [_ w236]
          tunnel: w125 -> [w235 _]
          tunnel: w105 -> [w231 _]
          tunnel: [w233 _] -> w124
          tunnel: [w232 w236] -> w70
          tunnel: w104 -> [w230 _]
          frame False {
            # "No [ClientName] \nEither SRTRS Office user OR\nCMS OR\nDB Error"
            n67 = call "DB - Replace DB.Schema.Table.vi"("DB.Schema.Table 2"=w230, "DB.Schema.Table"=w231, "string in"="USE [<DB>]\nSELECT \n     a.[PlantId]\n    ,a.[Description] as [Plant Description]\n    ,b.[StationId]\n    ,b.[Description] as [Station Description]\n    ,a.[DefaultLanguage] \n       \nFROM [<Schema>].[<Table>] as a\nRIGHT JOIN [<Schema2>].[<Table2>] as b\nON a.[PlantId] = b.[PlantId]\nWHERE a.[Inactive] = '0' AND\nb.[Inactive] = '0'  AND b.[ClientName] = 'GENERAL'\nORDER BY [PlantId] ASC") -> ("string out"=w233:string)  [unwired: 7 in, 1 out]
            n68 = call "DB - T-SQL Query.vi"("T-SQL"=w233, "connection reference"=w235) -> ("error out"=w229:errorcluster, "2D data"=w232:string[][])  [unwired: 7 in, 1 out]
            n69 = local write "DB Error"(w229) -> ()
          }
          frame True {
            # "[ClientName] Found"
          }
        }
        n70 = case shown="True" "Simulate DB Fail" {
          tunnel: w70 -> [w210 _]
          tunnel: [w210 w212] -> w69
          tunnel: w68 -> [w209 _]
          tunnel: [w209 FALSE] -> w67
          frame False {
          }
          frame True {
            w212 = string[][] []  # Blank Array (DB Fail)
          }
        }
        "2D data" <- w69
        "[ClientName] Found" <- w67
        n71 = Index Array(array=w69, index (row)=w153) -> (element=w100:string[])  [unwired: 1 in]
        n72 = Index Array(array=w69, index (col) #1=w84, index (col) #2=w99, index (col) #3=w93) -> (element #1=w83:string[], element #2=w87:string[], element #3=w86:string[])  [unwired: 3 in]
        n73 = Index Array(array=w100, index #1=w152, index #2=w151, index #3=w150, index #4=w149) -> (element #1=w78:string, element #2=w89:string, element #3=→"Station Description":string, element #4=w73:string)
        "[StationId]" <- w89
        "[PlantId]" <- w78
        n74 = Empty String/Path?(string/path=w73) -> (empty?=w76:bool)
        n75 = Build Array(w134, w133) -> (w132:string[][])
        n76 = Select(t="en", s=w76, f=w73) -> (s? t:f=→"[DefaultLanguage]":string)
        n77 = Index Array(array=w190, index (col) #1=w191, index (col) #2=w192) -> (element #1=w184:string[], element #2=w189:string[])  [unwired: 2 in]
        n78 = Transpose 2D Array(2D array=w132) -> (transposed array=→"[SpecialPrivilege] List":string[][])
        n79 = Index Array(array=w171, index (col) #1=w172, index (col) #2=w169, index (col) #3=w81) -> (element #1=w168:string[], element #2=w167:string[], element #3=w80:string[])  [unwired: 3 in]
        n80 = Empty String/Path?(string/path=w78) -> (empty?=w72:bool)
        n81 = call "DB - Convert BIT Type.vi"("BIT Type (eg Inactive) (Array)"=w189) -> ("Boolean (Array)"=w185:bool[])  [unwired: 2 in, 2 out]
        n82 = for {
          tunnel: w168 -> [w247] mode=indexing
          tunnel: w167 -> [w245] mode=indexing
          tunnel: [w248] -> w166 mode=indexing
          tunnel: w73 -> [w246]
          tunnel: [w245] -> w164 if=w244
          n83 = Equal?(x=w247, y=w246) -> (x = y?=w244:bool)
          n84 = Bundle(w247, w245) -> (w248:cluster{string, string})  [unwired: 1 in]
        }
        n85 = Not(x=w72) -> (.not. x?=w71:bool)
        "DB available" <- w71
        n86 = Index Array(array=w69, index (col) #1=w109, index (col) #2=w110) -> (element #1=w114:string[], element #2=w111:string[])  [unwired: 2 in]
        n87 = Search 1D Array(1D array=w185, element=TRUE) -> (index of element=w186:i32)  [unwired: 1 in]
        n88 = call "DB - Convert BIT Type.vi"("BIT Type (eg Inactive) (Array)"=w80) -> ("Boolean (Array)"=→"[IsUnicode]":bool[])  [unwired: 2 in, 2 out]
        n89 = Max & Min "if NOT FOUND (-1),\nwe set 0 (1st element)"(x=w186, y=0) -> (max(x,y)=w187:i32)  [unwired: 1 out]
        n90 = Index Array(array=w114, index=w115) -> (element=w82:string)
        n91 = for {
          tunnel: w83 -> [w220] mode=indexing
          tunnel: w82 -> [w219]
          tunnel: w87 -> [w218] mode=indexing
          tunnel: [w218] -> w88 mode=indexing if=w216
          tunnel: w86 -> [w217] mode=indexing
          tunnel: [w217] -> w85 mode=indexing if=w216
          n92 = Equal?(x=w220, y=w219) -> (x = y?=w216:bool)
        }
        n93 = call "String - Array Group By.vi"("Array in"=w114) -> ("GROUP BY (Array in)"=w113:string[])  [unwired: 10 in]
        n94 = call "String - Array Group By.vi"("Array in"=w111) -> ("GROUP BY (Array in)"=w112:string[])  [unwired: 10 in]
        n95 = call "String - Array Group By.vi"("Array in"=w88) -> ("GROUP BY (Array in)"=w92:string[])  [unwired: 10 in]
        n96 = call "String - Array Group By.vi"("Array in"=w85) -> ("GROUP BY (Array in)"=w91:string[])  [unwired: 10 in]
        n97 = local read "Application"() -> (w77:string)
        n98 = for {
          tunnel: w113 -> [w224] mode=indexing
          tunnel: w112 -> [w226] mode=indexing
          tunnel: [w228] -> w108 mode=indexing
          tunnel: w82 -> [w227]
          tunnel: [w226] -> w107 if=w225
          n99 = Equal?(x=w224, y=w227) -> (x = y?=w225:bool)
          n100 = Bundle("String"=w224, "String"=w226) -> (w228:cluster{"String":string, "String":string})  [unwired: 1 in]
        }
        n101 = Index Array(array=w184, index=w187) -> (element=w183:string)
        n102 = for {
          tunnel: w92 -> [w221] mode=indexing
          tunnel: w91 -> [w222] mode=indexing
          tunnel: [w223] -> w90 mode=indexing
          n103 = Bundle("String"=w221, "String"=w222) -> (w223:cluster{"String":string, "String":string})  [unwired: 1 in]
        }
        n104 = local write "Language (long form)"(w164) -> ()
        n105 = case shown="\"SRTRS\", Default" w77 {
          tunnel: w71 -> [w213 w214 w215]
          frame "CMS" {
            n106 = global write "Global CMS.vi" "DB Available"(w213) -> ()
          }
          frame "AMS" {
            n107 = global write "Global AMS.vi" "DB Available"(w214) -> ()
          }
          frame "SRTRS", Default {
            n108 = global write "Global SRTRS.vi" "DB Available"(w215) -> ()
          }
        }
        n109 = property on="Language" class="CmbBox (strict)"(error in=w62, "Strings And Values[]"=w166, "Value"=w73) -> (error out=w61:errorcluster)  [unwired: 1 in, 1 out]
        n110 = local write "Plant Description"(w107) -> ()
        n111 = property on="Plant" class="CmbBox (strict)"("Strings And Values[]"=w108, "Text.Text"=w82) -> ()  [unwired: 2 in, 2 out]
        n112 = property on="Station" class="CmbBox (strict)"("Text.Text"=w89, "Strings And Values[]"=w90) -> ()  [unwired: 2 in, 2 out]
        n113 = call "Logon - Module.vi"("Logon - Enum"=Logon_-_Enum."Check AD", "Logon User"="SRTRS") -> ("Error Out"=w130:errorcluster, "AD Info"=w161:T14)  [unwired: 4 in, 4 out]
        n114 = local write "Logon Error"(w130) -> ()
        n115 = local write "DB Error"(w61) -> ()
        n116 = Unbundle By Name(w161) -> ("AD available"=w159:bool)
        n117 = Build Array(w123, w124, w154, w170, w145) -> (w202:string[])
        n118 = case shown="\"Disable Simulation\", Default" "AD Simulate" {
          tunnel: w159 -> [_ _ w243]
          tunnel: [TRUE FALSE ("AD available") w243] -> w158
          frame "Simulate AD Available" {
          }
          frame "Simulate AD NOT Available" {
          }
          frame "Disable Simulation", Default {
          }
        }
        "AD available" <- w158
        n119 = case shown="False" w158 {
          tunnel: w184 -> [_ w240]
          tunnel: w183 -> [_ w239]
          tunnel: ["LOCAL" w239] -> w157
          tunnel: [_ w238] -> w156
          frame False {
            # "AD Not Avaliable"
          }
          frame True {
            # "AD Available"
            n120 = property on="Domain" class="CmbBox (strict)"("Strings[]"=w240) -> (error out=w238:errorcluster)  [unwired: 2 in, 1 out]
          }
        }
        n121 = property on="Domain" class="CmbBox (strict)"(error in=w156, "Value"=w157) -> ()  [unwired: 1 in, 2 out]
      }
      event "Logon Button": Value Change {
        w275 = 28  # [Stations]
        w276 = 27  # [AllStations]
        w286 = 6  # [RawDataReport]
        w289 = 7  # b.[Tab0]
        w314 = 2  # [Password]
        w297 = 5  # [SpecialPrivilege]
        w315 = 0  # [UserName]
        # "User Has Access if DB Fails"
        n122 = event-data() -> ("CtlRef"=w293:refnum<vi>)  [unwired: 1 in, 5 out]
        n123 = To Upper Case(1:"Domain") -> (0:w299:T5)
        n124 = call "Logon - Module.vi"("Logon - Enum"=Logon_-_Enum."Check AD", "Logon User"="SRTRS") -> ("AD Info"=w305:T14)  [unwired: 4 in, 5 out]
        n125 = local read "AD Simulate"() -> (w303:T3)
        n126 = Unbundle By Name(w305) -> ("AD available"=w304:bool)
        n127 = call "DB - Split DB.Schema.Table.vi"("DB.Schema.Table"="DB.Config.UserStationAccess") -> ("DB.Schema.Table"=w278:T12)  [unwired: 10 in]
        n128 = call "DB - Split DB.Schema.Table.vi"("DB.Schema.Table"="DB.Config.TabUserAccess") -> ("DB.Schema.Table"=w290:T12)  [unwired: 10 in]
        n129 = call "DB - Split DB.Schema.Table.vi"("DB.Schema.Table"="DB.Admin.Users") -> ("DB.Schema.Table"=w333:T12)  [unwired: 10 in]
        n130 = case shown="\"Disable Simulation\"" w303 {
          tunnel: w304 -> [_ _ w439]
          tunnel: [TRUE FALSE ("AD available") w439] -> w302
          frame "Simulate AD Available", Default {
          }
          frame "Simulate AD NOT Available" {
          }
          frame "Disable Simulation" {
          }
        }
        n131 = call "DB - Replace DB.Schema.Table.vi"("DB.Schema.Table 3"=w278, "DB.Schema.Table 2"=w290, "DB.Schema.Table"=w333, "string in"="USE [<DB>]\nSELECT TOP 1\n  a.[UserName] \n  ,a.[DomainId]\n  ,a.[Password]\n  ,a.[TabAccessId]\n  ,a.[StationAccessId]\n  ,a.[SpecialPrivilege]\n  ,a.[RawDataReport]\n  \n  ,b.[Tab0] ,b.[Tab1] ,b.[Tab2]  ,b.[Tab3] ,b.[Tab4] \n ,b.[Tab5] ,b.[Tab6] ,b.[Tab7]  ,b.[Tab8] ,b.[Tab9] \n ,b.[Tab10] ,b.[Tab11] ,b.[Tab12]  ,b.[Tab13] ,b.[Tab14] \n ,b.[Tab15] ,b.[Tab16] ,b.[Tab17]  ,b.[Tab18] ,b.[Tab19]\n\n ,c.[AllStations]\n ,c.[Stations]\n\nFROM [<Schema>].[<Table>] AS a\nLEFT JOIN [<Schema2>].[<Table2>] AS b\nON \na.[PlantId] = b.[PlantId] AND\n a.[TabAccessId] = b.[TabAccessId]\nLEFT JOIN [<Schema3>].[<Table3>] as c\nON\na.[PlantId] = c.[PlantId] AND\na.[StationAccessId] = c.[StationAccessId] \n\nWHERE \na.[PlantId] = '<A>' AND\na.[UserId] = '<B>' AND\na.[Inactive] = '0' AND\nb.[Inactive] = '0' AND\nc.[Inactive] = '0'\n") -> ("string out"=w326:string)  [unwired: 6 in, 1 out]
        n132 = property on="Plant" class="CmbBox (strict)"() -> ("Text.Text"=w321:string)  [unwired: 2 in, 2 out]
        n133 = Search and Replace String(input string=w326, search string="<A>" ("input string"), replace string=w321) -> (result string=w324:string)  [unwired: 5 in, 3 out]
        n134 = local read "User"() -> (w313:string)
        n135 = Search and Replace String(input string=w324, search string="<B>" ("input string"), replace string=w313) -> (result string=w312:string)  [unwired: 5 in, 3 out]
        n136 = call-poly <vilib>:"DB Tools Execute Query.vi"("error in (no error)"=w320, "SQL query"=w312, "connection reference"=w300) -> ("error out"=w330:errorcluster, "recordset reference"=w331:T13)  [unwired: 5 in]
        n137 = call-poly <vilib>:"DB Tools Fetch Recordset Data.vi"("error in (no error)"=w330, "recordset reference"=w331) -> ("error out"=w329:errorcluster, "recordset data"=w323:variant[][], "recordset reference out"=w332:T13)  [unwired: 3 in]
        n138 = local write "AD available"(w302) -> ()
        n139 = call-poly <vilib>:"DB Tools Free Object.vi"("error in (no error)"=w329, "recordset reference"=w332) -> ("error out"=w319:errorcluster)  [unwired: 8 in, 1 out]
        n140 = local read "DB available"() -> (w252:bool)
        n141 = Variant To Data(error in=w319, type=string[][] [], Variant=w323) -> (data=w317:string[][], error out=w267:errorcluster)
        n142 = local write "DB Error"(w267) -> ()
        n143 = Index Array(array=w317, index (row)=0) -> (element=w277:string[])  [unwired: 1 in]
        n144 = flat-sequence {
          tunnel: w254 -> [_]
          tunnel: [""] -> w253
          frame #0 {
            n145 = property on="Station" class="CmbBox (strict)"() -> ("Text.Text"=w336:string)  [unwired: 2 in, 2 out]
            n146 = property on="Plant" class="CmbBox (strict)"() -> ("Text.Text"=w337:string)  [unwired: 2 in, 2 out]
            n147 = global read "Global AMS.vi" "Logon"() -> (w340:T1)
            n148 = global read "Global SRTRS.vi" "Logon"() -> (w338:T1)
            n149 = global read "Global CMS.vi" "Logon"() -> (w341:T1)
            n150 = Bundle By Name(cluster=w341, "PlantID"=w337, "StationID"=w336) -> (w342:T1)
            n151 = Bundle By Name(cluster=w340, "PlantID"=w337, "StationID"=w336) -> (w339:T1)
            n152 = Bundle By Name(cluster=w338, "PlantID"=w337, "StationID"=w336) -> (w335:T1)
            n153 = global write "Global CMS.vi" "Logon"(w342) -> ()
            n154 = global write "Global AMS.vi" "Logon"(w339) -> ()
            n155 = global write "Global SRTRS.vi" "Logon"(w335) -> ()
          }
        }
        n156 = Array Size(array=w277) -> (size(s)=w308:i32)
        n157 = Index Array(array=w277, index #1=w315, index #2=w314, index #3=w297, index #4=w286) -> (element #1=→"[UserName]":string, element #2=w254:string, element #3=w296:string, element #4=w285:string)
        n158 = Index Array(array=w277, index #1=w276, index #2=w275) -> (element #1=w274:string, element #2=w273:string)
        n159 = call "DB - Convert BIT Type.vi"("BIT Type (eg Inactive)"=w296) -> ("Boolean"=w309:bool)  [unwired: 2 in, 2 out]
        n160 = case shown="\"LOCAL\"" w299 {
          tunnel: w302 -> [_ w444]
          tunnel: w309 -> [_ w443]
          tunnel: w308 -> [_ w442]
          tunnel: [DB_-_Logon_Authentication_Enum."AD Authentication" w441] -> w251
          frame "False", Default {
            # "NOT Local Domain"
          }
          frame "LOCAL" {
            # "LOCAL Domain"
            n161 = case shown="True" w444 {
              tunnel: w443 -> [_ w448]
              tunnel: w442 -> [_ w447]
              tunnel: [DB_-_Logon_Authentication_Enum."Local Authentication" w446] -> w441
              frame False {
                # "AD Not Available"
              }
              frame True {
                # "AD Available"
                n162 = case shown="True" w448 {
                  tunnel: w447 -> [_ w451]
                  tunnel: [DB_-_Logon_Authentication_Enum."NO Authentication" w450] -> w446
                  frame False {
                    # "NOT [SpecialPrivilege]"
                  }
                  frame True {
                    # "[SpecialPrivilege]"
                    n163 = case shown="0" w451 {
                      tunnel: [DB_-_Logon_Authentication_Enum."NO Authentication" DB_-_Logon_Authentication_Enum."Local Authentication"] -> w450
                      frame 0 {
                        # "No Records Found.\nLocal Authentication FAIL"
                      }
                      frame 1, Default {
                        # "Record Found\nPerform Local Authentication"
                      }
                    }
                  }
                }
              }
            }
          }
        }
        n164 = Select(t=w251, s=w252, f=DB_-_Logon_Authentication_Enum."NODB Authentication") -> (s? t:f=w250:T11)
        n165 = case shown="\"NODB Authentication\"" w250 {
          tunnel: [w399 w410 FALSE w430] -> w261
          tunnel: ["" w418 "" ""] -> w301
          tunnel: w254 -> [_ w417 _ _]
          tunnel: w300 -> [_ w416 _ _]
          tunnel: w299 -> [w401 _ _ _]
          frame "AD Authentication", Default {
            # "Used by {Logon} only, stores the RSSLogon.exe file"
            # "AD Authentication is DONE here\n(Both Server & Local)"
            n166 = call "Logon - Module.vi"("Main Application Directory"="Main Application Directory (SRTRS/CMS/AMS)", "Logon - Enum"=Logon_-_Enum."Logon", "Password"="Password", "Domain"=w401, "Logon User"="User") -> ("Error Out"=→"Logon Error":errorcluster, "Logon OK"=w399:bool)  [unwired: 1 in, 4 out]
            n167 = case shown="False" w399 {
              tunnel: "User" -> [_ w407]
              frame False {
              }
              frame True {
                n168 = call "Logon - Module.vi"("Logon - Enum"=Logon_-_Enum."Check AD", "Logon User"=w407) -> ("Error Out"=w404:errorcluster, "AD Info"=w406:T14)  [unwired: 4 in, 4 out]
                n169 = local write "Logon Error"(w404) -> ()
                n170 = Unbundle By Name(w406) -> ("Logon Full Name"=w405:string)
                n171 = local write "[UserName]"(w405) -> ()
              }
            }
          }
          frame "Local Authentication" {
            # "DB OK"
            # "SELECT HASHBYTES('MD4', @HashThis);"
            # "If DB Fails, there will be NO Local Authentication"
            n172 = local read "DB Error"() -> (w409:errorcluster)
            n173 = local read "Password"() -> (w424:string)
            n174 = Search and Replace String(input string="SELECT CONVERT(nvarchar(32) ,HASHBYTES('MD4', '<C>'),2)" ("string"), search string="<C>", replace string=w424) -> (result string=w418:string)  [unwired: 5 in, 3 out]
            n175 = call-poly <vilib>:"DB Tools Execute Query.vi"("error in (no error)"=w409, "SQL query"=w418, "connection reference"=w416) -> ("error out"=w419:errorcluster, "recordset reference"=w420:T13)  [unwired: 5 in]
            n176 = call-poly <vilib>:"DB Tools Fetch Element Data.vi"("error in (no error)"=w419, "column index"=0, "recordset reference"=w420) -> ("error out"=w425:errorcluster, "data"=w414:string, "recordset reference out"=w426:T13)  [unwired: 4 in]
            n177 = call-poly <vilib>:"DB Tools Free Object.vi"("error in (no error)"=w425, "recordset reference"=w426) -> ("error out"=w415:errorcluster)  [unwired: 8 in, 1 out]
            n178 = String Length(string=w414) -> (length=w413:i32)
            n179 = Equal?(x=w417, y=w414) -> (x = y?=w411:bool)
            n180 = local write "DB Error"(w415) -> ()
            n181 = Greater Than 0?(x=w413) -> (x > 0?=w412:bool)
            n182 = And(x=w411, y=w412) -> (x .and. y?=w410:bool)
          }
          frame "NO Authentication" {
          }
          frame "NODB Authentication" {
            n183 = local read "User"() -> (w435:string)
            n184 = local read "Password"() -> (w433:string)
            n185 = Equal?(x=w435, y="NODB") -> (x = y?=w432:bool)
            n186 = Equal?(x=w433, y="Password") -> (x = y?=w431:bool)
            n187 = And(x=w432, y=w431) -> (x .and. y?=w430:bool)
          }
        }
        n188 = call "DB - Convert BIT Type.vi"("BIT Type (eg Inactive)"=w285) -> ("Boolean"=→"[RawDataReport]":bool)  [unwired: 2 in, 2 out]
        n189 = call "DB - Convert BIT Type.vi"("BIT Type (eg Inactive)"=w274) -> ("Boolean"=w269:bool)  [unwired: 2 in, 2 out]
        "[AllStations]" <- w269
        n190 = Array Subset(array=w277, index=w289, length=20) -> (w287:string[])
        n191 = Spreadsheet String To Array(delimiter (Tab)=",", format string="", spreadsheet string=w273, array type (2D Dbl)=string[] []) -> (array=w268:string[])
        "[Stations]" <- w268
        n192 = flat-sequence {
          tunnel: w293 -> [w373]
          tunnel: [w373] -> w292
          frame #0 {
            # "Toggle Effect on Button"
            n193 = Wait (ms)(milliseconds to wait=u32 100) -> ()  [unwired: 1 out]
          }
        }
        n194 = call "DB - Convert BIT Type.vi"("BIT Type (eg Inactive) (Array)"=w287) -> ("Boolean (Array)"=→"[TabUserAccess]":bool[])  [unwired: 2 in, 2 out]
        n195 = case shown="False" w269 {
          selector: w269 -> [_ w367]
          tunnel: w268 -> [w366 _]
          tunnel: [w363 w367] -> w265
          frame False {
            n196 = property on="Station" class="CmbBox (strict)"() -> ("Text.Text"=w365:string)  [unwired: 2 in, 2 out]
            n197 = Search 1D Array(1D array=w366, element=w365) -> (index of element=w364:i32)  [unwired: 1 in]
            n198 = Greater Or Equal To 0?(x=w364) -> (x >= 0?=w363:bool)
          }
          frame True {
          }
        }
        "User Has Access" <- w265
        n199 = flat-sequence {
          tunnel: w259 -> [_]
          tunnel: w292 -> [w376]
          frame #0 {
            n200 = property class="Bool (strict)"(reference=w376, "Value"=FALSE) -> ()  [unwired: 1 in, 2 out]
          }
        }
        n201 = Select(t=TRUE, s=w267, f=w265) -> (s? t:f=w262:bool)
        n202 = case shown="True" w261 {
          tunnel: ["<E 102>" w352] -> w264
          tunnel: [_ w351] -> w263
          tunnel: w262 -> [_ w350]
          tunnel: [_ w349] -> w260
          tunnel: [_ w348] -> w259
          tunnel: ["Logon Failed" ("Short Description (When DB Not Available)") w347] -> w258
          tunnel: ["Invalid username or password. Please retry." ("Short Description (When DB Not Available)") w346] -> w257
          tunnel: w253 -> [_ _]
          frame False {
            # "Authentication Failed"
          }
          frame True {
            # "Authentication OK"
            n203 = case shown="True" w350 {
              tunnel: ["<E 106>" "<I 101>"] -> w352
              tunnel: [w356 w361] -> w351
              tunnel: [w355 _] -> w349
              tunnel: [_ TRUE] -> w348
              tunnel: ["Logon Failed." ("Short Description (When DB Not Available)") "Logon Successful" ("Short Description (When DB Not Available)")] -> w347
              tunnel: [" not authorized for this station." ("Short Description (When DB Not Available)") " logon successful." ("Short Description (When DB Not Available)")] -> w346
              frame False {
                # "User No Access"
                n204 = local read "Plant"() -> (w355:T5)
                n205 = local read "User"() -> (w356:string)
              }
              frame True {
                # "User has Access"
                n206 = local read "User"() -> (w361:string)
              }
            }
          }
        }
        "Logon PASS" <- w259
        n207 = case shown="True" w259 {
          tunnel: [w378 w393] -> w282
          tunnel: T1 {"PlantID"="", "SystemID"="", "UserID"="", "DomainID"="", "LanguageID"="", "StationID"=""} ("Login Constant") -> [w378 w392]
          tunnel: [w377 w389] -> w281
          tunnel: T2 {"Plant Name"="", "UserName"="", "Hostname [ClientName]"="", "IsUnicode"=FALSE} ("Logon Extra") -> [w377 w388]
          frame False {
          }
          frame True {
            n208 = local read "[IsUnicode]"() -> (w381:bool[])
            n209 = property on="Language" class="CmbBox (strict)"() -> ("Text.Text"=w382:string, "Strings[]"=w383:string[])  [unwired: 2 in, 2 out]
            n210 = local read "Plant Description"() -> (w391:string)
            n211 = local read "[UserName]"() -> (w390:string)
            n212 = local read "Hostname [ClientName]"() -> (w384:string)
            n213 = property on="Plant" class="CmbBox (strict)"() -> ("Text.Text"=w387:string)  [unwired: 2 in, 2 out]
            n214 = Search 1D Array(1D array=w383, element=w382) -> (index of element=w380:i32)  [unwired: 1 in]
            n215 = property on="Station" class="CmbBox (strict)"() -> ("Text.Text"=w386:string)  [unwired: 2 in, 2 out]
            n216 = local read "User"() -> (w395:string)
            n217 = local read "Domain"() -> (w394:T5)
            n218 = Index Array(array=w381, index=w380) -> (element=w379:bool)
            n219 = Bundle By Name(cluster=w388, "IsUnicode"=w379, "Plant Name"=w391, "UserName"=w390, "Hostname [ClientName]"=w384) -> (w389:T2)
            n220 = Bundle By Name(cluster=w392, "PlantID"=w387, "SystemID"="", "UserID"=w395, "DomainID"=w394, "LanguageID"=w382, "StationID"=w386) -> (w393:T1)
          }
        }
        n221 = flat-sequence {
          tunnel: w259 -> [_]
          frame #0 {
            n222 = local write "Password"("") -> ()
          }
        }
        n223 = Build Array(w312, w301) -> (w311:string[])
        n224 = local read "Application"() -> (w255:string)
        n225 = call "Msgbox - Message Handler.vi"("Application (Default SRTRS)"=w255, "Short Description (When DB Not Available)"=w258, "Description (When DB Not Available)"=w257, "Post-Description"=w260, "Pre-Description"=w263, "<.?....> Message Code"=w264) -> ("MHandler Error"=→"MHandler":errorcluster)  [unwired: 3 in, 2 out]
        n226 = flat-sequence "Logon OK last to be written because of VI Ref Read Loop" {
          tunnel: w282 -> [w368]
          tunnel: w281 -> [w370]
          tunnel: w259 -> [w369]
          tunnel: [w369] -> w280
          tunnel: w280 -> [w372]
          frame #0 {
            "Logon Extra" <- w370
            "Logon" <- w368
          }
          frame #1 {
            n227 = local write "Logon OK"(w372) -> ()
            n228 = local write "User"("") -> ()
          }
        }
      }
      event "Password": Key Down {
        n229 = event-data() -> ("VKey"=w455:T15)  [unwired: 1 in, 9 out]
        n230 = case shown="\"Enter\", \"Return\"" w455 {
          frame "ASCII", Default {
          }
          frame "Enter", "Return" {
            n231 = property on="Logon Button" class="Bool (strict)"("Val(Sgnl)"=TRUE) -> ()  [unwired: 2 in, 2 out]
          }
        }
      }
      event "Reinehold": Value Change {
        n232 = event-data() -> ()  [unwired: 1 in, 6 out]
        n233 = flat-sequence {
          frame #0 {
            n234 = local write "Password"("Welcome1973" ("Password")) -> ()
            n235 = local write "User"("Admin" ("User")) -> ()
            n236 = property on="Domain" class="CmbBox (strict)"("Value"="Local") -> ()  [unwired: 2 in, 2 out]
          }
          frame #1 {
            n237 = property on="Logon Button" class="Bool (strict)"("Val(Sgnl)"=TRUE) -> ()  [unwired: 2 in, 2 out]
          }
        }
      }
      event Value Change {
        n238 = event-data() -> ("CtlRef"=w464:refnum<vi>)  [unwired: 1 in, 5 out]
        n239 = property class="CmbBox (strict)"(reference=w464) -> ("Value"=w463:T5, "Label.Text"=w462:string, "Text.Text"=w461:string)  [unwired: 1 in, 2 out]
        n240 = case shown="\"Plant\", Default" w462 {
          tunnel: w463 -> [w478 w491]
          tunnel: w461 -> [w474 _]
          frame "Plant", Default {
            w470 = 3  # Station [Description]
            w473 = 2  # [StationId]
            w476 = 0  # [PlantId]
            # "Change Station Drop Down Option.\nWe do not Change Plant Drop Down if Station Changes. \nOnly 1 rule"
            # "[PlantId] can only change to a valid PlantId tied to [ClientName] during Initial check"
            # "[PlantId] has changed"
            n241 = local read "Plant Description"() -> (w480:string)
            n242 = local read "2D data"() -> (w477:string[][])
            n243 = Not Equal?(x=w480, y=w478) -> (x != y?=w479:bool)
            n244 = case shown="True" w479 {
              tunnel: w478 -> [_ w490]
              frame False {
              }
              frame True {
                w489 = ""
                # "Only Blanks out Station if Plant Changed"
                n245 = local write "Plant Description"(w490) -> ()
                n246 = local write "Station Description"(w489) -> ()
                n247 = property on="Station" class="CmbBox (strict)"("Text.Text"=w489) -> ()  [unwired: 2 in, 2 out]
              }
            }
            n248 = Index Array(array=w477, index (col) #1=w476, index (col) #2=w473, index (col) #3=w470) -> (element #1=w475:string[], element #2=w472:string[], element #3=w469:string[])  [unwired: 3 in]
            n249 = for {
              tunnel: w475 -> [w488] mode=indexing
              tunnel: w474 -> [w487]
              tunnel: w472 -> [w486] mode=indexing
              tunnel: [w486] -> w471 mode=indexing if=w484
              tunnel: w469 -> [w485] mode=indexing
              tunnel: [w485] -> w468 mode=indexing if=w484
              n250 = Equal?(x=w488, y=w487) -> (x = y?=w484:bool)
            }
            n251 = call "String - Array Group By.vi"("Array in"=w468) -> ("GROUP BY (Array in)"=w466:string[])  [unwired: 10 in]
            n252 = call "String - Array Group By.vi"("Array in"=w471) -> ("GROUP BY (Array in)"=w467:string[])  [unwired: 10 in]
            n253 = for {
              tunnel: w467 -> [w481] mode=indexing
              tunnel: w466 -> [w482] mode=indexing
              tunnel: [w483] -> w465 mode=indexing
              n254 = Bundle("String"=w481, "String"=w482) -> (w483:cluster{"String":string, "String":string})  [unwired: 1 in]
            }
            n255 = property on="Station" class="CmbBox (strict)"("Strings And Values[]"=w465) -> ()  [unwired: 2 in, 2 out]
          }
          frame "Station" {
            n256 = local write "Station Description"(w491) -> ()
          }
        }
      }
      event Value Change {
        n257 = event-data() -> ("NewVal"=w493:T5)  [unwired: 1 in, 5 out]
        n258 = To Upper Case(1:w493) -> (0:w492:T5)
        n259 = Equal?(x=w492, y="LOCAL") -> (x = y?=w494:bool)
        n260 = case shown="True" w494 {
          frame False {
          }
          frame True {
            # "Check if Special USER"
            n261 = local read "[SpecialPrivilege] List"() -> (w506:string[][])
            n262 = property on="Plant" class="CmbBox (strict)"() -> ("Text.Text"=w496:string)  [unwired: 2 in, 2 out]
            n263 = local read "User"() -> (w504:string)
            n264 = Index Array(array=w506, index (col) #1=0 ("disabled index (col)"), index (col) #2=1 ("index (col)")) -> (element #1=w501:string[], element #2=w500:string[])  [unwired: 2 in]
            n265 = Concatenate Strings(w496, w504) -> (w503:string)
            n266 = for {
              tunnel: w501 -> [w512] mode=indexing
              tunnel: w500 -> [w511] mode=indexing
              tunnel: [w510] -> w499 mode=indexing
              n267 = Concatenate Strings(w512, w511) -> (w510:string)
            }
            n268 = Search 1D Array(1D array=w499, element=w503) -> (index of element=w497:i32)  [unwired: 1 in]
            n269 = Greater Or Equal To 0?(x=w497) -> (x >= 0?=w498:bool)
            n270 = local read "AD available"() -> (w509:bool)
            n271 = Not(x=w509) -> (.not. x?=w508:bool)
            n272 = Or(x=w498, y=w508) -> (x .or. y?=w507:bool)
            n273 = case shown="False" w507 {
              frame False {
                # "NOT special User\nCheck if AD available. If AD Available, use CCC. Cannot use Local."
                n274 = local read "AD Simulate"() -> (w515:T3)
                n275 = call "Logon - Module.vi"("Logon - Enum"=Logon_-_Enum."PC username") -> ("Error Out"=w516:errorcluster, "AD Info"=w518:T14)  [unwired: 5 in, 4 out]
                n276 = Unbundle By Name(w518) -> ("PC username"=w517:string)
                n277 = call "Logon - Module.vi"("Logon - Enum"=Logon_-_Enum."Check AD", "Error In"=w516, "Logon User"=w517) -> ("AD Info"=w520:T14)  [unwired: 3 in, 5 out]
                n278 = Unbundle By Name(w520) -> ("AD available"=w514:bool)
                n279 = case shown="\"Simulate AD NOT Available\"" w515 {
                  tunnel: w514 -> [_ _ w524]
                  tunnel: [TRUE FALSE ("AD available") w524] -> w513
                  frame "Simulate AD Available", Default {
                  }
                  frame "Simulate AD NOT Available" {
                  }
                  frame "Disable Simulation" {
                  }
                }
                n280 = local write "AD available"(w513) -> ()
                n281 = case shown="True" w513 {
                  frame False {
                  }
                  frame True {
                    # "AD available\nReset Domain"
                    n282 = local read "Application"() -> (w525:string)
                    n283 = local write "Domain"("CCC") -> ()
                    n284 = call "Msgbox - Message Handler.vi"("Application (Default SRTRS)"=w525, "<.?....> Message Code"="<E 103>") -> ("MHandler Error"=w526:errorcluster)  [unwired: 7 in, 2 out]
                    n285 = local write "MHandler"(w526) -> ()
                  }
                }
              }
              frame True {
                # "Special USER\nCan use any Domain"
              }
            }
          }
        }
      }
      event Value Change {
        n286 = event-data() -> ()  [unwired: 1 in, 6 out]
        n287 = property on="Language" class="CmbBox (strict)"() -> ("Value"=→"Language (long form)":T5)  [unwired: 2 in, 2 out]
      }
    }
    "Error Out" <- w57
    "SQL" <- w56
  }
  n288 = call <vilib>:"DB Tools Close Connection.vi"("error in (no error)"=w2, "connection reference"=w4) -> ("error out"=w1:errorcluster)  [unwired: 5 in]
  n289 = local write "DB Error"(w1) -> ()
